vi "Read OOIs.vi"(8 "error in (no error)":errorcluster, 9 "File Path Control":path=path "D:/Espen Tolpinrud/My Documents/LabView/AUR Control System/ROV/Configuration", 10 "ROV Selector":u16(ring) items=["Minerva", "Neptune"], 11 "Vessel In":refnum<class "Vessel.lvclass">) -> (0 "error out":errorcluster, 1 "Observer Names":string[](array[string]), 2 "Controller Names":string[](array[string]), 3 "Vessel Out":refnum<class "Vessel.lvclass">)   [LabVIEW 2012, in "Vessel.lvclass"]
doc: "This method reads a configuration file with a predefined setup in xml. The system is then configured accordingly such that all sensors are initialized, observers and controllers are tuned and all values are given."
uses:
  Vessel.lvclass
  Vessel.lvclass/Vessel.ctl
  <vilib>/LabVIEW Targets/FPGA/cRIO/shared/nicrio_ModuleControls/nicrio_cRIO-9871_FlowControlEnum.ctl
  <vilib>/LabVIEW Targets/FPGA/cRIO/shared/nicrio_ModuleControls/nicrio_cRIO-9871_BaudRateEnum.ctl
  <vilib>/LabVIEW Targets/FPGA/cRIO/shared/nicrio_ModuleControls/nicrio_cRIO-9871_DataBitsEnum.ctl
  <vilib>/LabVIEW Targets/FPGA/cRIO/shared/nicrio_ModuleControls/nicrio_cRIO-9871_ParityEnum.ctl
  <vilib>/LabVIEW Targets/FPGA/cRIO/shared/nicrio_ModuleControls/nicrio_cRIO-9871_StopBitsEnum.ctl
  Observer/Kalman Filter/Kalman Filter.lvclass
  Observer/Attitude Observer/Attitude Observer.lvclass
  Observer/HG Observer/HG Observer.lvclass
  Joystick/Joystick Guidance.lvclass
  Guidance/Altitude Guidance/Altitude Guidance.lvclass
  Guidance/Constant Jerk Guidance/Constant Jerk Guidance.lvclass
  Guidance/CJ Switcher/CJ switcher.lvclass
  Controller/PID Controller/Non Linear PID Controller/Non Linear PID Controller.lvclass
  <vilib>/xml/Load XML File.vi
  Sensor/Sensor(StringArray).vi
  <vilib>/Analysis/Matrix/Numeric/Multiply/Multiply - RM,R.vi
  Observer/Kalman Filter Altitude/Kalman Filter Altitude().vi
  Observer/Kalman Filter/Kalman Filter (Vessel).vi
  Observer/HG Observer/HG Observer().vi
  Joystick/Joystick Guidance ().vi
  Guidance/Constant Jerk Guidance/CJ Guidance().vi
  Controller/PID Controller/Non Linear PID Controller/Non Linear PID Controller().vi
  Thruster/Thruster(ArrayInput).vi
  <resource>/objmgr/DOMUserDefRef.rc
  <vilib>/xml/NI_XML.lvlib
  Sensor/Sensor.lvclass
  Thrust Allocation/Thrust Allocation.lvclass
  Thruster/Thruster.lvclass
  Observer/Kalman Filter Altitude/Kalman Filter Altitude.lvclass
  Controller/Controller.lvclass
  <vilib>/Analysis/Matrix/NI_Matrix.lvlib
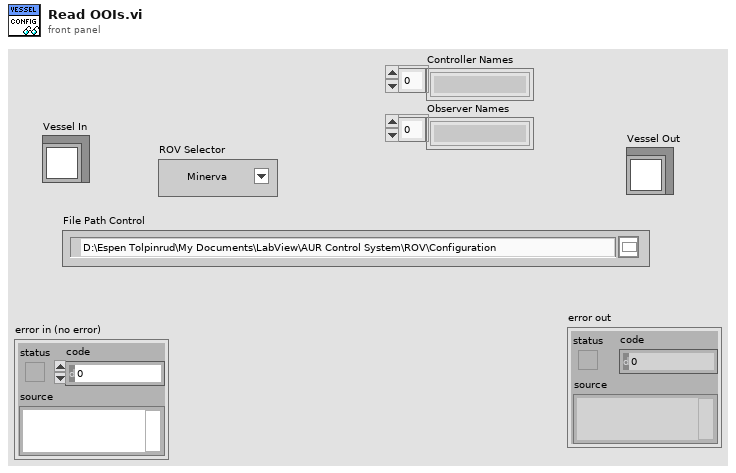
[diagram p1: front panel]
types:
  T1 = typedef "nicrio_cRIO-9871_FlowControlEnum.ctl" = enum8{"None", "Software (XON / XOFF)", "Hardware (RTS / CTS)"}
  T2 = typedef "nicrio_cRIO-9871_StopBitsEnum.ctl" = enum8{"1", "1.5", "2"}
  T3 = typedef "nicrio_cRIO-9871_DataBitsEnum.ctl" = enum8{"5", "6", "7", "8"}
  T4 = typedef "nicrio_cRIO-9871_ParityEnum.ctl" = enum8{"None", "Odd", "Even", "Mark", "Space"}
  T5 = typedef "nicrio_cRIO-9871_BaudRateEnum.ctl" = enum16{"75 bps", "110 bps", "134 bps", "150 bps", "300 bps", "600 bps", "1200 bps", "1800 bps", "2400 bps", "4800 bps", "7200 bps", "9600 bps", "14.4 kbps", "19.2 kbps", "28.8 kbps", "38.4 kbps", "57.6 kbps", "115.2 kbps", "230.4 kbps", "460.8 kbps", "921.6 kbps"}
  T6 = cluster{"Baud Rate":T5, "Data Bits":T3, "Parity":T4, "Stop Bits":T2, "Flow Control":T1}[]
  T7 = cluster{"Baud Rate":T5, "Data Bits":T3, "Parity":T4, "Stop Bits":T2, "Flow Control":T1}
  T8 = typedef "NI_Matrix.lvlib/RealMatrix.ctl" = dbl[][]
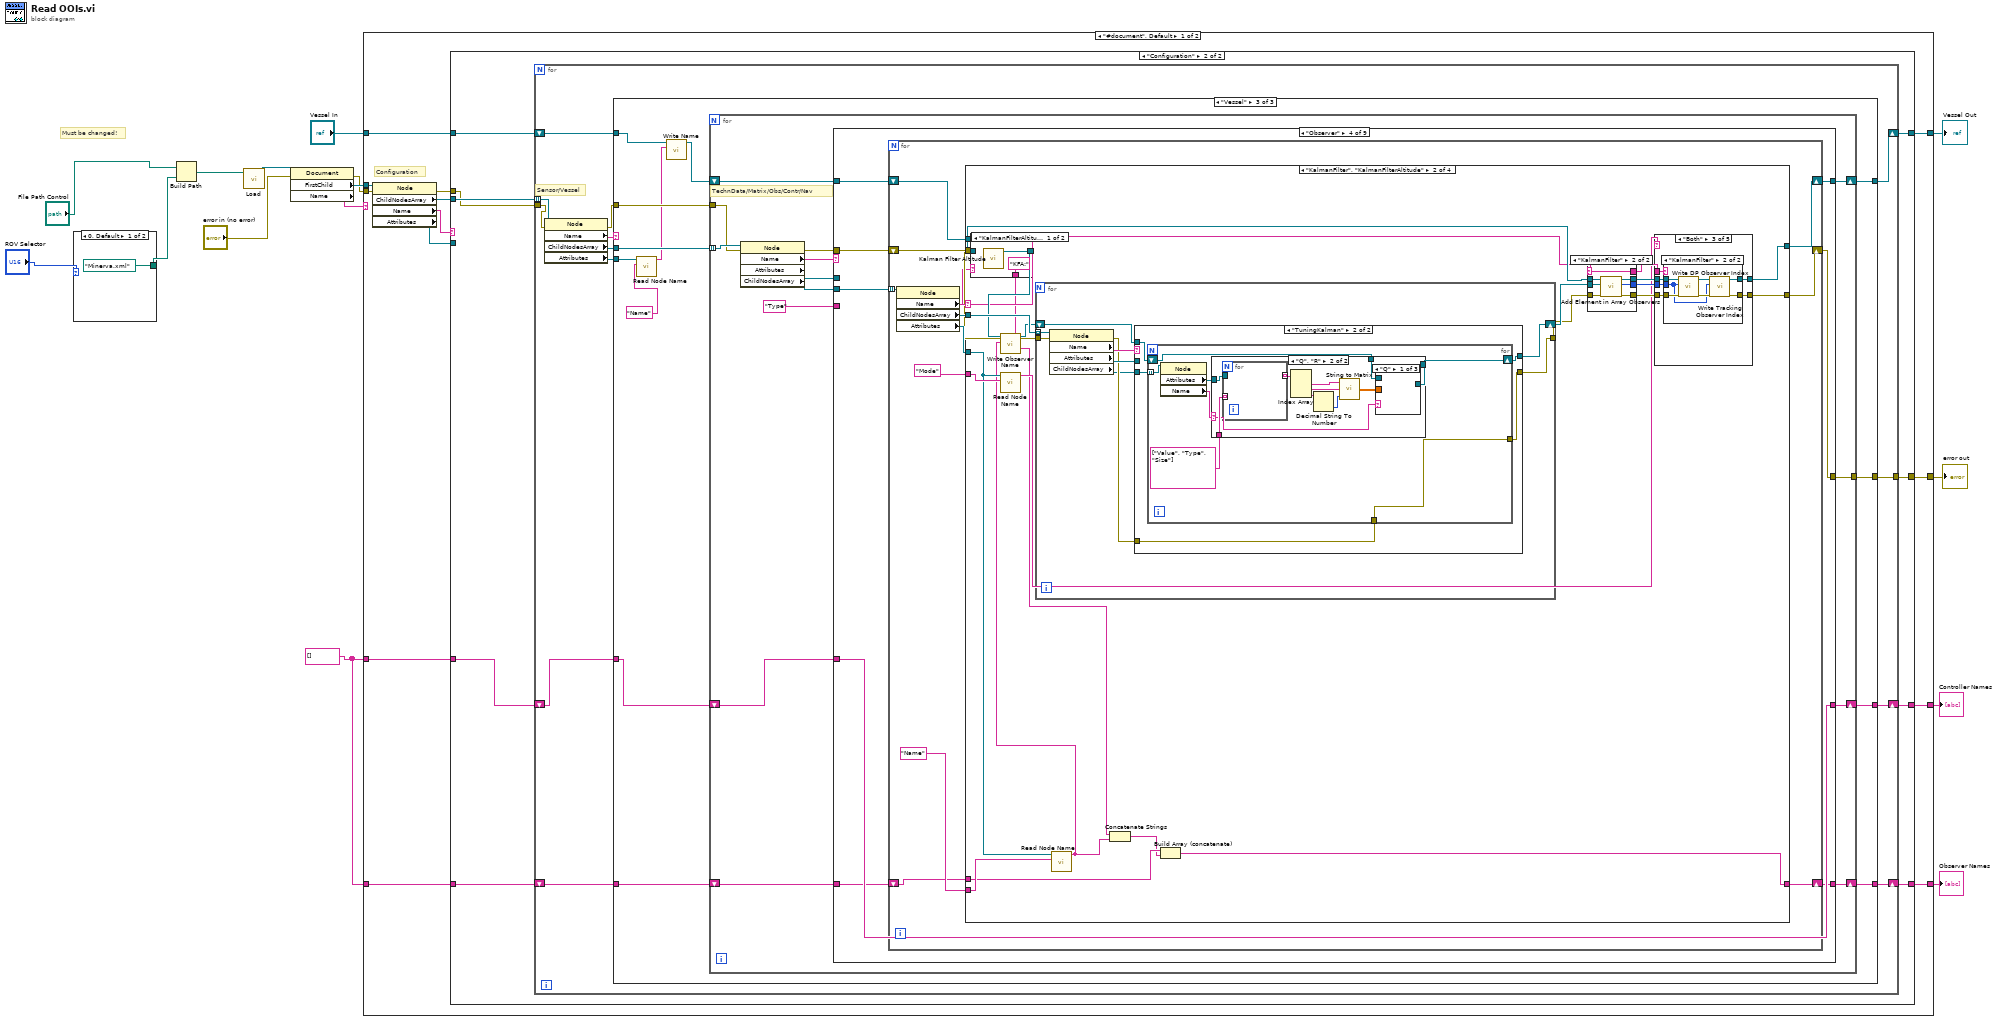
[diagram p0: block diagram]
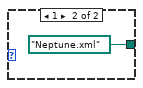
[diagram p2: hidden frame]
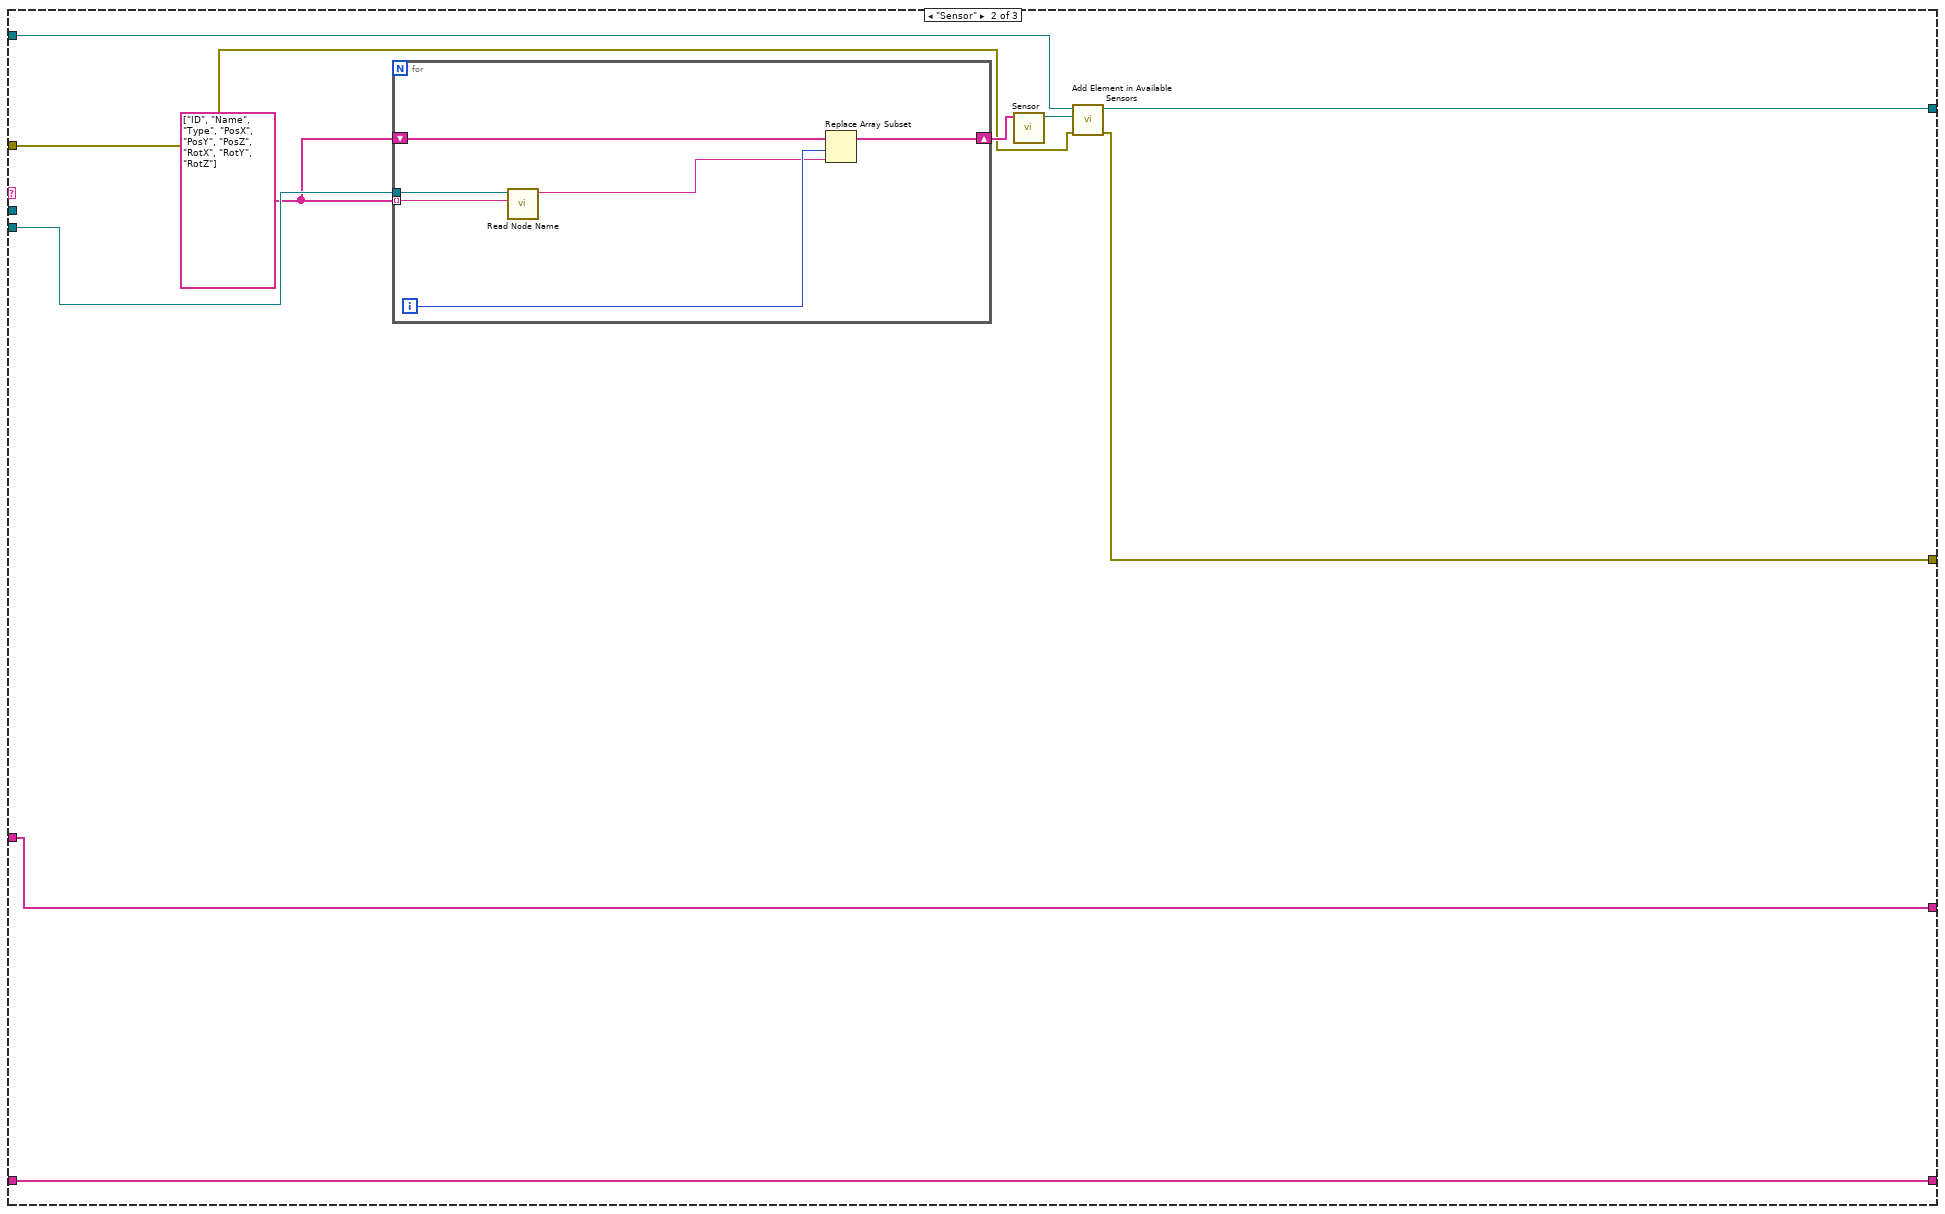
[diagram p5: hidden frame]
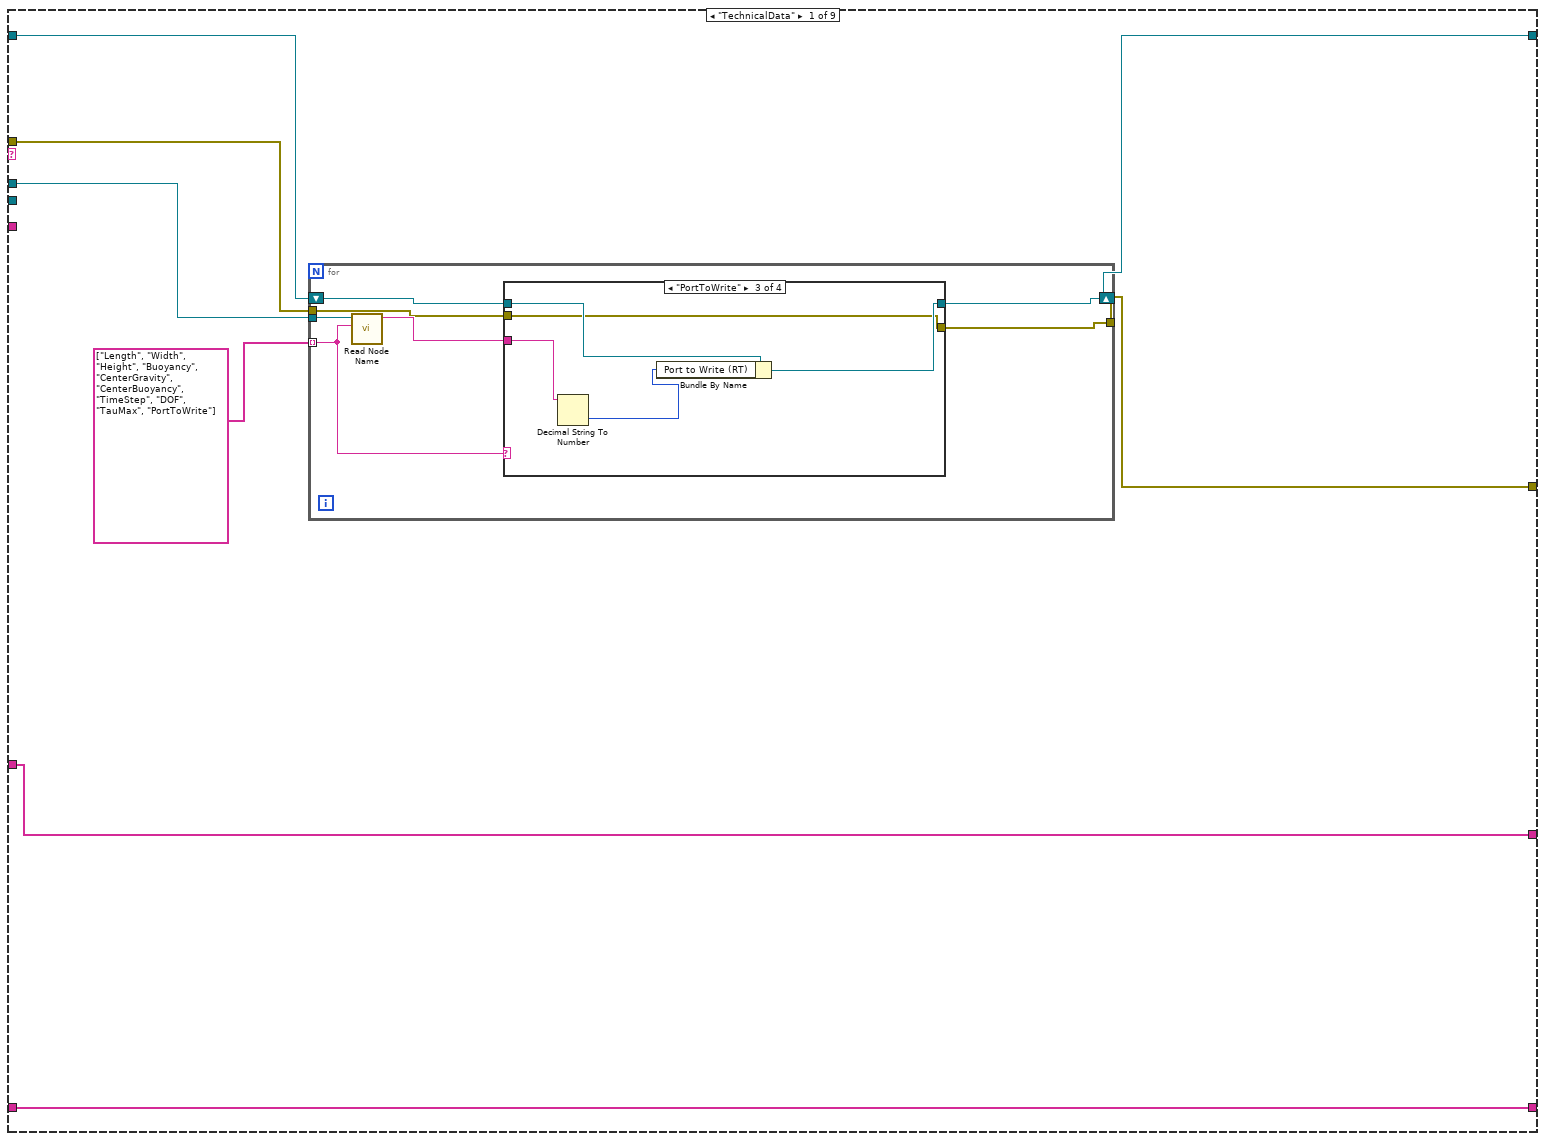
[diagram p6: hidden frame]
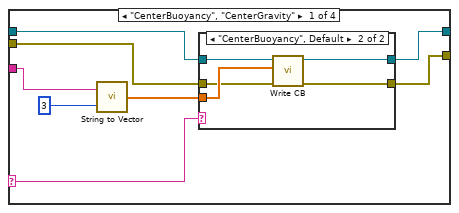
[diagram p7: hidden frame]
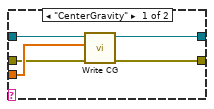
[diagram p8: hidden frame]
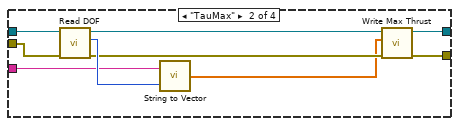
[diagram p9: hidden frame]
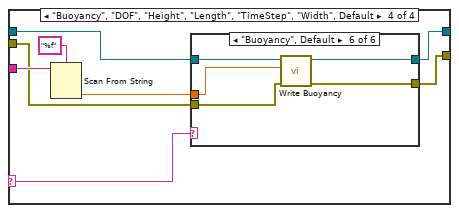
[diagram p10: hidden frame]
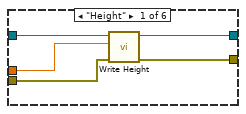
[diagram p11: hidden frame]
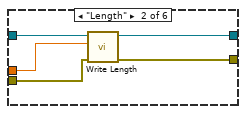
[diagram p12: hidden frame]
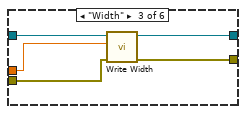
[diagram p13: hidden frame]
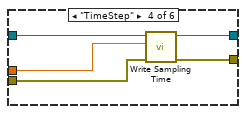
[diagram p14: hidden frame]
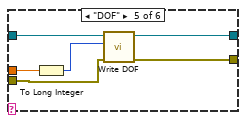
[diagram p15: hidden frame]
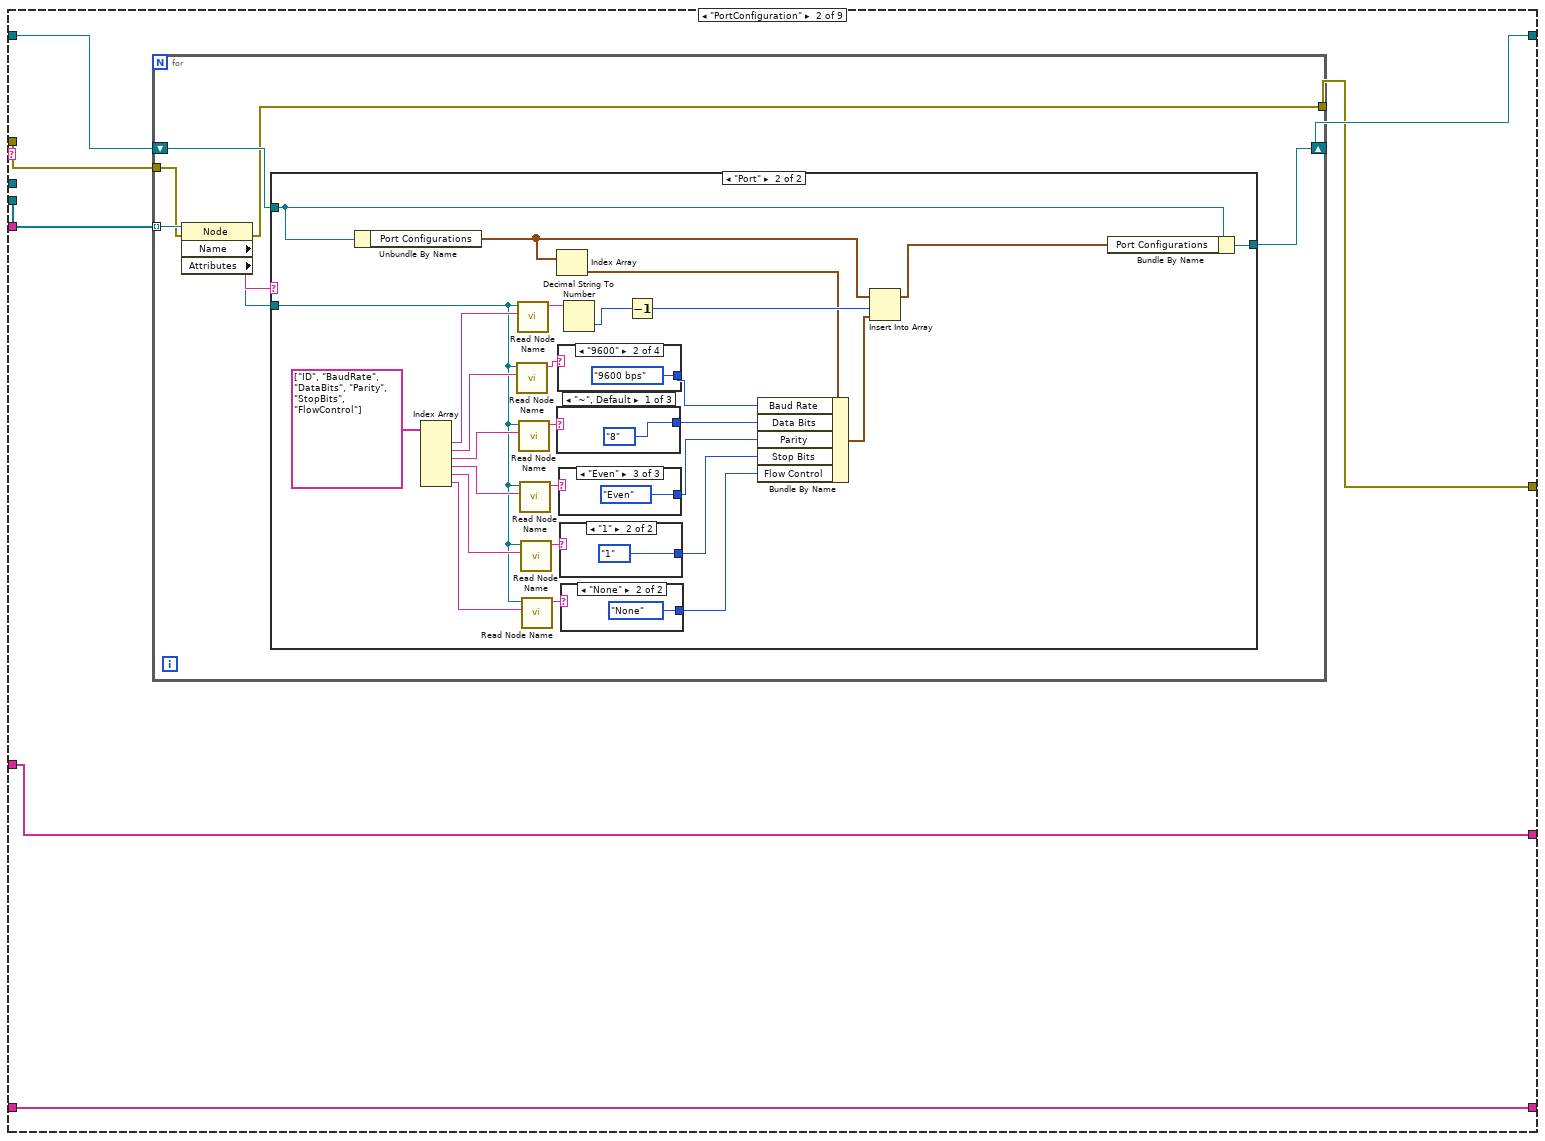
[diagram p16: hidden frame]
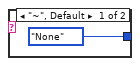
[diagram p18: hidden frame]
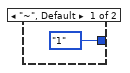
[diagram p19: hidden frame]
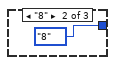
[diagram p20: hidden frame]
diagram:
  w2 = string[] []
  # "Must be changed!"
  n1 = case shown="0, Default" "ROV Selector" {
    tunnel: [path "Minerva.xml" path "Neptune.xml"] -> w6
    frame 0, Default {
    }
    frame 1 {
    }
  }
  n2 = Build Path(base path="File Path Control", name or relative path=w6) -> (appended path=w5:path)
  n3 = call-poly <vilib>:"Load.vi"("path to XML document"=w5) -> ("DOM document out"=w15:refnum<k20>)  [unwired: 12 in, 2 out]
  n4 = property class="Document"(reference=w15, error in="error in (no error)") -> (error out=w10:errorcluster, "FirstChild"=w14:refnum<k20>, "Name"=w13:string)  [unwired: 1 out]
  n5 = case shown="\"#document\", Default" w13 {
    tunnel: w14 -> [w30 _]
    tunnel: "Vessel In" -> [w26 w1002]
    tunnel: [w25 w1002] -> w11
    tunnel: w10 -> [w24 w1001]
    tunnel: [w22 w1001] -> w8
    tunnel: [w21 w1000] -> w3
    tunnel: w2 -> [w20 w1000]
    tunnel: w2 -> [w19 w999]
    tunnel: [w18 w999] -> w1
    frame "#document", Default {
      # "Configuration"
      n6 = property class="Node"(reference=w30, error in=w24) -> (error out=w23:errorcluster, "ChildNodesArray"=w27:refnum<k20>[], "Name"=w28:string, "Attributes"=w29:refnum<k20>)  [unwired: 1 out]
      n7 = case shown="\"Configuration\"" w28 {
        tunnel: w29 -> [_ _]
        tunnel: w27 -> [_ w43]
        tunnel: w26 -> [w34 w42]
        tunnel: [w34 w41] -> w25
        tunnel: w23 -> [w33 w40]
        tunnel: [w33 w39] -> w22
        tunnel: [w32 w38] -> w21
        tunnel: w20 -> [w32 w37]
        tunnel: w19 -> [w31 w36]
        tunnel: [w31 w35] -> w18
        frame "#~", Default {
        }
        frame "Configuration" {
          n8 = for {
            tunnel: w43 -> [w56] mode=indexing
            tunnel: w40 -> [w52]
            tunnel: [w50] -> w39
            shift-right: [w48] -> w41
            shift-left: w42 -> [w49]
            shift-right: [w47] -> w38
            shift-left: w37 -> [w46]
            shift-right: [w44] -> w35
            shift-left: w36 -> [w45]
            # "Sensor/Vessel"
            n9 = property class="Node"(reference=w56, error in=w52) -> (error out=w51:errorcluster, "Name"=w55:string, "ChildNodesArray"=w54:refnum<k20>[], "Attributes"=w53:refnum<k20>)  [unwired: 1 out]
            n10 = case shown="\"Vessel\"" w55 {
              tunnel: w54 -> [_ _ w89]
              tunnel: w53 -> [_ w70 w85]
              tunnel: w49 -> [w60 w67 w83]
              tunnel: [w60 w66 w88] -> w48
              tunnel: w51 -> [w59 w65 w87]
              tunnel: [w59 w63 w86] -> w50
              tunnel: [w58 w62 w80] -> w47
              tunnel: w46 -> [w58 w62 w79]
              tunnel: w45 -> [w57 w61 w78]
              tunnel: [w57 w61 w77] -> w44
              frame "#~", Default {
              }
              frame "Sensor" {
                w64 = string[] ["ID", "Name", "Type", "PosX", "PosY", "PosZ", "RotX", "RotY", "RotZ"]
                n11 = for {
                  tunnel: w64 -> [w73] mode=indexing
                  tunnel: w70 -> [w74]
                  shift-right: [w75] -> w69
                  shift-left: w64 -> [w71]
                  i -> [w76]
                  n12 = call "Read Node Name.vi"("Name"=w73, "Attributes"=w74) -> ("Value"=w72:string)  [unwired: 9 in]
                  n13 = Replace Array Subset(array=w71, new element=w72, index=w76) -> (w75:string[])
                }
                n14 = call-poly "Sensor.vi"("Input"=w69) -> ("Sensor.lvclass"=w68:refnum<class "Sensor.lvclass">)  [unwired: 10 in]
                n15 = call "Add Element in Available Sensors.vi"("error in (no error)"=w65, "Sensor In"=w68, "Vessel in"=w67) -> ("error out"=w63:errorcluster, "Vessel out"=w66:refnum<class "Vessel.lvclass">)  [unwired: 7 in]
              }
              frame "Vessel" {
                n16 = call "Read Node Name.vi"("Name"="Name", "Attributes"=w85) -> ("Value"=w84:string)  [unwired: 9 in]
                n17 = call-dynamic "Write Name.vi"("Name"=w84, "Vessel in"=w83) -> ("Vessel out"=w82:refnum<class "Vessel.lvclass">)  [unwired: 8 in, 1 out]
                n18 = for {
                  tunnel: w89 -> [w103] mode=indexing
                  tunnel: w87 -> [w98]
                  tunnel: [w96] -> w86
                  shift-right: [w95] -> w88
                  shift-left: w82 -> [w94]
                  shift-right: [w93] -> w80
                  shift-left: w79 -> [w92]
                  shift-right: [w90] -> w77
                  shift-left: w78 -> [w91]
                  # "TechnData/Matrix/Obs/Contr/Nav"
                  n19 = property class="Node"(reference=w103, error in=w98) -> (error out=w97:errorcluster, "Name"=w102:string, "Attributes"=w101:refnum<k20>, "ChildNodesArray"=w100:refnum<k20>[])  [unwired: 1 out]
                  n20 = case shown="\"Observer\"" w102 {
                    tunnel: w101 -> [w111 _ _ _ _ w764 w918 w978 _]
                    tunnel: w100 -> [_ w196 w249 w313 w586 w768 _ _ _]
                    tunnel: w94 -> [w109 w195 w252 w310 w584 w767 w915 w972 w998]
                    tunnel: [w108 w194 w251 w311 w583 w763 w917 w971 w998] -> w95
                    tunnel: "Type" -> [_ _ _ _ _ _ w920 _ _]
                    tunnel: w97 -> [w107 w193 w250 w312 w585 w766 w916 w970 w997]
                    tunnel: [w106 w192 w248 w309 w582 w765 w914 w969 w997] -> w96
                    tunnel: [w105 w191 w247 w308 w581 w762 w913 w968 w996] -> w93
                    tunnel: w92 -> [w105 w191 w247 w308 w581 w761 w913 w968 w996]
                    tunnel: w91 -> [w104 w190 w246 w307 w580 w760 w912 w967 w995]
                    tunnel: [w104 w190 w246 w306 w580 w760 w912 w967 w995] -> w90
                    frame "TechnicalData" {
                      n21 = for {
                        tunnel: w111 -> [w118]
                        tunnel: string[] ["Length", "Width", "Height", "Buoyancy", "CenterGravity", "CenterBuoyancy", "TimeStep", "DOF", "TauMax", "PortToWrite"] -> [w117] mode=indexing
                        shift-right: [w114] -> w108
                        shift-left: w109 -> [w115]
                        tunnel: w107 -> [w113]
                        tunnel: [w112] -> w106
                        n22 = call "Read Node Name.vi"("Name"=w117, "Attributes"=w118) -> ("Value"=w116:string)  [unwired: 9 in]
                        n23 = case shown="\"PortToWrite\"" w117 {
                          selector: w117 -> [w126 _ _ w155]
                          tunnel: w116 -> [w123 w141 w149 w158]
                          tunnel: w115 -> [w125 w144 w150 w156]
                          tunnel: [w124 w145 w148 w153] -> w114
                          tunnel: w113 -> [w120 w140 w147 w152]
                          tunnel: [w119 w138 w147 w151] -> w112
                          frame "CenterBuoyancy", "CenterGravity" {
                            n24 = call "String to Vector.vi"("Vector Dimension"=3, "String Input"=w123) -> ("Vector"=w122:dbl[])
                            n25 = case shown="\"CenterBuoyancy\", Default" w126 {
                              tunnel: w125 -> [w131 w136]
                              tunnel: [w130 w135] -> w124
                              tunnel: w122 -> [w129 w134]
                              tunnel: w120 -> [w128 w133]
                              tunnel: [w127 w132] -> w119
                              frame "CenterGravity" {
                                n26 = call "Write CG.vi"("error in (no error)"=w128, "CG"=w129, "Vessel in"=w131) -> ("error out"=w127:errorcluster, "Vessel out"=w130:refnum<class "Vessel.lvclass">)  [unwired: 7 in]
                              }
                              frame "CenterBuoyancy", Default {
                                n27 = call "Write CB.vi"("error in (no error)"=w133, "CB"=w134, "Vessel in"=w136) -> ("error out"=w132:errorcluster, "Vessel out"=w135:refnum<class "Vessel.lvclass">)  [unwired: 7 in]
                              }
                            }
                          }
                          frame "TauMax" {
                            n28 = call-dynamic "Read DOF.vi"("error in (no error)"=w140, "Vessel in"=w144) -> ("error out"=w139:errorcluster, "DOF"=w142:i32, "Vessel out"=w143:refnum<class "Vessel.lvclass">)  [unwired: 7 in]
                            n29 = call "String to Vector.vi"("Vector Dimension"=w142, "String Input"=w141) -> ("Vector"=w137:dbl[])
                            n30 = call "Write Max Thrust.vi"("error in (no error)"=w139, "Max Thrust"=w137, "Vessel in"=w143) -> ("error out"=w138:errorcluster, "Vessel out"=w145:refnum<class "Vessel.lvclass">)  [unwired: 7 in]
                          }
                          frame "PortToWrite" {
                            n31 = Decimal String To Number(string=w149) -> (number=w146:i32)  [unwired: 2 in, 1 out]
                            n32 = Bundle By Name(cluster=w150, "Port to Write (RT)"=w146) -> (w148:refnum<class "Vessel.lvclass">)
                          }
                          frame "Buoyancy", "DOF", "Height", "Length", "TimeStep", "Width", Default {
                            n33 = Scan From String(format string="%f", input string=w158) -> (output 1=w154:dbl)  [unwired: 3 in, 3 out]
                            n34 = case shown="\"Buoyancy\", Default" w155 {
                              tunnel: w156 -> [w163 w168 w173 w178 w184 w189]
                              tunnel: w154 -> [w161 w167 w171 w176 w182 w187]
                              tunnel: [w162 w166 w172 w177 w183 w188] -> w153
                              tunnel: w152 -> [w160 w165 w170 w175 w180 w186]
                              tunnel: [w159 w164 w169 w174 w179 w185] -> w151
                              frame "Height" {
                                n35 = call-dynamic "Write Height.vi"("error in (no error)"=w160, "Height"=w161, "Vessel in"=w163) -> ("error out"=w159:errorcluster, "Vessel out"=w162:refnum<class "Vessel.lvclass">)  [unwired: 7 in]
                              }
                              frame "Length" {
                                n36 = call-dynamic "Write Length.vi"("error in (no error)"=w165, "Length"=w167, "Vessel in"=w168) -> ("error out"=w164:errorcluster, "Vessel out"=w166:refnum<class "Vessel.lvclass">)  [unwired: 7 in]
                              }
                              frame "Width" {
                                n37 = call-dynamic "Write Width.vi"("error in (no error)"=w170, "Width"=w171, "Vessel in"=w173) -> ("error out"=w169:errorcluster, "Vessel out"=w172:refnum<class "Vessel.lvclass">)  [unwired: 7 in]
                              }
                              frame "TimeStep" {
                                n38 = call-dynamic "Write Sampling Time.vi"("error in (no error)"=w175, "Sampling Time"=w176, "Vessel in"=w178) -> ("error out"=w174:errorcluster, "Vessel out"=w177:refnum<class "Vessel.lvclass">)  [unwired: 7 in]
                              }
                              frame "DOF" {
                                n39 = To Long Integer(number=w182) -> (32bit integer=w181:i32)
                                n40 = call-dynamic "Write DOF.vi"("error in (no error)"=w180, "DOF"=w181, "Vessel in"=w184) -> ("error out"=w179:errorcluster, "Vessel out"=w183:refnum<class "Vessel.lvclass">)  [unwired: 7 in]
                              }
                              frame "Buoyancy", Default {
                                n41 = call-dynamic "Write Buoyancy.vi"("error in (no error)"=w186, "Buoyancy"=w187, "Vessel in"=w189) -> ("error out"=w185:errorcluster, "Vessel out"=w188:refnum<class "Vessel.lvclass">)  [unwired: 7 in]
                              }
                            }
                          }
                        }
                      }
                    }
                    frame "PortConfiguration" {
                      n42 = for {
                        tunnel: w196 -> [w203] mode=indexing
                        shift-right: [w199] -> w194
                        shift-left: w195 -> [w200]
                        tunnel: w193 -> [w198]
                        tunnel: [w197] -> w192
                        n43 = property class="Node"(reference=w203, error in=w198) -> (error out=w197:errorcluster, "Name"=w202:string, "Attributes"=w201:refnum<k20>)  [unwired: 1 out]
                        n44 = case shown="\"Port\"" w202 {
                          tunnel: w201 -> [_ w224]
                          tunnel: w200 -> [w204 w217]
                          tunnel: [w204 w215] -> w199
                          frame "#~", Default {
                          }
                          frame "Port" {
                            n45 = Unbundle By Name(w217) -> ("Port Configurations"=w220:T6)
                            n46 = Index Array(array=string[] ["ID", "BaudRate", "DataBits", "Parity", "StopBits", "FlowControl"]) -> (element #1=w230:string, element #2=w229:string, element #3=w228:string, element #4=w227:string, element #5=w226:string, element #6=w225:string)  [unwired: 6 in]
                            n47 = call "Read Node Name.vi"("Name"=w229, "Attributes"=w224) -> ("Value"=w214:string)  [unwired: 9 in]
                            n48 = call "Read Node Name.vi"("Name"=w230, "Attributes"=w224) -> ("Value"=w223:string)  [unwired: 9 in]
                            n49 = call "Read Node Name.vi"("Name"=w228, "Attributes"=w224) -> ("Value"=w210:string)  [unwired: 9 in]
                            n50 = call "Read Node Name.vi"("Name"=w227, "Attributes"=w224) -> ("Value"=w212:string)  [unwired: 9 in]
                            n51 = call "Read Node Name.vi"("Name"=w226, "Attributes"=w224) -> ("Value"=w208:string)  [unwired: 9 in]
                            n52 = call "Read Node Name.vi"("Name"=w225, "Attributes"=w224) -> ("Value"=w206:string)  [unwired: 9 in]
                            n53 = Index Array(array=w220) -> (element=w219:T7)  [unwired: 1 in]
                            n54 = case shown="\"~\", Default" w210 {
                              tunnel: [nicrio_cRIO-9871_DataBitsEnum."8" ("Data Bits") nicrio_cRIO-9871_DataBitsEnum."8" ("Data Bits") nicrio_cRIO-9871_DataBitsEnum."7" ("Data Bits")] -> w209
                              frame "~", Default {
                              }
                              frame "8" {
                              }
                              frame "7" {
                              }
                            }
                            n55 = case shown="\"9600\"" w214 {
                              tunnel: [nicrio_cRIO-9871_BaudRateEnum."57.6 kbps" ("Baud Rate") nicrio_cRIO-9871_BaudRateEnum."9600 bps" ("Baud Rate") nicrio_cRIO-9871_BaudRateEnum."115.2 kbps" ("Baud Rate") nicrio_cRIO-9871_BaudRateEnum."19.2 kbps" ("Baud Rate")] -> w213
                              frame "57.6", Default {
                              }
                              frame "9600" {
                              }
                              frame "115.2" {
                              }
                              frame "19.2" {
                              }
                            }
                            n56 = case shown="\"Even\"" w212 {
                              tunnel: [nicrio_cRIO-9871_ParityEnum."None" ("Parity") nicrio_cRIO-9871_ParityEnum."None" ("Parity") nicrio_cRIO-9871_ParityEnum."Even" ("Parity")] -> w211
                              frame "~", Default {
                              }
                              frame "None" {
                              }
                              frame "Even" {
                              }
                            }
                            n57 = case shown="\"1\"" w208 {
                              tunnel: [nicrio_cRIO-9871_StopBitsEnum."1" ("Stop Bits") nicrio_cRIO-9871_StopBitsEnum."1" ("Stop Bits")] -> w207
                              frame "~", Default {
                              }
                              frame "1" {
                              }
                            }
                            n58 = case shown="\"None\"" w206 {
                              tunnel: [nicrio_cRIO-9871_FlowControlEnum."None" ("Flow Control") nicrio_cRIO-9871_FlowControlEnum."None" ("Flow Control")] -> w205
                              frame "~", Default {
                              }
                              frame "None" {
                              }
                            }
                            n59 = Decimal String To Number(string=w223) -> (number=w222:i32)  [unwired: 2 in, 1 out]
                            n60 = Decrement(x=w222) -> (x-1=w221:i32)
                            n61 = Bundle By Name(cluster=w219, "Baud Rate"=w213, "Data Bits"=w209, "Parity"=w211, "Stop Bits"=w207, "Flow Control"=w205) -> (w218:T7)
                            n62 = Insert Into Array(array=w220, index=w221, new element=w218) -> (w216:T6)
                            n63 = Bundle By Name(cluster=w217, "Port Configurations"=w216) -> (w215:refnum<class "Vessel.lvclass">)
                          }
                        }
                      }
                    }
                    frame "Matrix" {
                      n64 = for {
                        tunnel: w249 -> [w262] mode=indexing
                        tunnel: w250 -> [w259]
                        tunnel: [w258] -> w248
                        shift-right: [w253] -> w251
                        shift-left: w252 -> [w254]
                        n65 = property class="Node"(reference=w262, error in=w259) -> (error out=w255:errorcluster, "Name"=w257:string, "Attributes"=w260:refnum<k20>)  [unwired: 1 out]
                        n66 = case shown="\"AddedMass\", \"Corriolis\", \"LinearDamping\", \"Mass\", \"NonLinearDamping\"" w257 {
                          selector: w257 -> [w264 w271]
                          tunnel: [dbl[][] [] w265] -> w261
                          tunnel: w260 -> [_ w269]
                          tunnel: [w264 w271] -> w256
                          frame "#~", Default {
                          }
                          frame "AddedMass", "Corriolis", "LinearDamping", "Mass", "NonLinearDamping" {
                            n67 = call "Read Node Name.vi"("Name"="Values", "Attributes"=w269) -> ("Value"=w266:string)  [unwired: 9 in]
                            n68 = call "Read Node Name.vi"("Name"="Size", "Attributes"=w269) -> ("Value"=w274:string)  [unwired: 9 in]
                            n69 = call "Read Node Name.vi"("Name"="Type", "Attributes"=w269) -> ("Value"=w268:string)  [unwired: 9 in]
                            n70 = Decimal String To Number(string=w274) -> (number=w267:i32)  [unwired: 2 in, 1 out]
                            n71 = call "String to Matrix.vi"("Matrix Size"=w267, "Matrix Type"=w268, "Value string"=w266) -> ("Output Matrix"=w265:T8)
                          }
                        }
                        n72 = case shown="\"NonLinearDamping\"" w256 {
                          tunnel: w261 -> [_ w278 w286 w293 w296 w303]
                          tunnel: w254 -> [w276 w283 w288 w292 w300 w305]
                          tunnel: [w276 w282 w287 w291 w299 w304] -> w253
                          tunnel: w255 -> [w275 w281 w285 w290 w298 w302]
                          tunnel: [w275 w280 w284 w289 w297 w301] -> w258
                          frame "#~", Default {
                          }
                          frame "Mass" {
                            n73 = call-poly <vilib>:"Multiply.vi"("Real Scalar c"=1, "Real Matrix A"=w278) -> ("A * c"=w277:T8)
                            n74 = call "Write Mass_RB.vi"("error in (no error)"=w281, "Real Matrix"=w277, "Vessel in"=w283) -> ("error out"=w280:errorcluster, "Vessel out"=w282:refnum<class "Vessel.lvclass">)  [unwired: 7 in]
                          }
                          frame "AddedMass" {
                            n75 = call "Write Mass_A.vi"("error in (no error)"=w285, "Real Matrix"=w286, "Vessel in"=w288) -> ("error out"=w284:errorcluster, "Vessel out"=w287:refnum<class "Vessel.lvclass">)  [unwired: 7 in]
                          }
                          frame "LinearDamping" {
                            n76 = call "Write Linear Damping.vi"("error in (no error)"=w290, "Real Matrix"=w293, "Vessel in"=w292) -> ("error out"=w289:errorcluster, "Vessel out"=w291:refnum<class "Vessel.lvclass">)  [unwired: 7 in]
                          }
                          frame "NonLinearDamping" {
                            n77 = call-poly <vilib>:"Multiply.vi"("Real Scalar c"=1, "Real Matrix A"=w296) -> ("A * c"=w294:T8)
                            n78 = call "Write Nonlinear Damping.vi"("error in (no error)"=w298, "Real Matrix"=w294, "Vessel in"=w300) -> ("error out"=w297:errorcluster, "Vessel out"=w299:refnum<class "Vessel.lvclass">)  [unwired: 7 in]
                          }
                          frame "Corriolis" {
                            n79 = call "Write Coriolis_RB.vi"("error in (no error)"=w302, "Real Matrix"=w303, "Vessel in"=w305) -> ("error out"=w301:errorcluster, "Vessel out"=w304:refnum<class "Vessel.lvclass">)  [unwired: 7 in]
                          }
                        }
                      }
                    }
                    frame "Observer" {
                      n80 = for {
                        tunnel: w313 -> [w322] mode=indexing
                        shift-right: [w324] -> w311
                        shift-left: w310 -> [w323]
                        shift-right: [w317] -> w309
                        shift-left: w312 -> [w325]
                        shift-right: [w315] -> w306
                        shift-left: w307 -> [w314]
                        n81 = property class="Node"(reference=w322) -> ("Name"=w321:string, "ChildNodesArray"=w320:refnum<k20>[], "Attributes"=w318:refnum<k20>)  [unwired: 1 in, 2 out]
                        n82 = case shown="\"KalmanFilter\", \"KalmanFilterAltitude\"" w321 {
                          selector: w321 -> [_ w336 _ _]
                          tunnel: w325 -> [w328 w351 w480 w542]
                          tunnel: w323 -> [w327 w346 w481 w545]
                          tunnel: [w327 w348 w479 w544] -> w324
                          tunnel: w320 -> [_ w341 w484 w554]
                          tunnel: "Mode" -> [_ w340 _ _]
                          tunnel: w318 -> [_ w334 w477 w548]
                          tunnel: [w328 w347 w480 w541] -> w317
                          tunnel: "Name" -> [_ w335 w478 w547]
                          tunnel: [w326 w332 w475 w546] -> w315
                          tunnel: w314 -> [w326 w333 w476 w549]
                          frame "#~", Default {
                          }
                          frame "KalmanFilter", "KalmanFilterAltitude" {
                            n83 = case shown="\"KalmanFilterAltitude\", Default" w336 {
                              tunnel: [w423 w426] -> w337
                              tunnel: w346 -> [_ w425]
                              tunnel: ["KFA:" "KFR:"] -> w329
                              frame "KalmanFilterAltitude", Default {
                                n84 = call-poly "Kalman Filter Altitude.vi"() -> ("Kalman Filter Altitude Out"=w423:refnum<class "Kalman Filter Altitude.lvclass">)  [unwired: 11 in]
                              }
                              frame "KalmanFilter" {
                                n85 = call-poly "Kalman Filter.vi"("Vessel.lvclass"=w425) -> ("Observer Library.lvlib:Kalman Filter.lvclass"=w426:refnum<class "Kalman Filter.lvclass">)  [unwired: 10 in]
                              }
                            }
                            n86 = call "Read Node Name.vi"("Name"=w340, "Attributes"=w334) -> ("Value"=w339:string)  [unwired: 9 in]
                            n87 = call "Read Node Name.vi"("Name"=w335, "Attributes"=w334) -> ("Value"=w331:string)  [unwired: 9 in]
                            n88 = call-dynamic "Write Observer Name.vi"("Observer Name"=w331, "Observer in"=w337) -> ("Observer out"=w338:refnum<class "Kalman Filter.lvclass">)  [unwired: 8 in, 1 out]
                            n89 = for {
                              tunnel: w341 -> [w435] mode=indexing
                              tunnel: [w428] -> w349
                              tunnel: w351 -> [w432]
                              shift-right: [w431] -> w350
                              shift-left: w338 -> [w430]
                              n90 = property class="Node"(reference=w435, error in=w432) -> (error out=w429:errorcluster, "Name"=w434:string, "Attributes"=w433:refnum<k20>, "ChildNodesArray"=w427:refnum<k20>[])  [unwired: 1 out]
                              n91 = case shown="\"TuningKalman\"" w434 {
                                tunnel: w433 -> [_ _]
                                tunnel: [w437 w439] -> w431
                                tunnel: w430 -> [w437 w440]
                                tunnel: w429 -> [w436 w442]
                                tunnel: [w436 w438] -> w428
                                tunnel: w427 -> [_ w441]
                                frame "#~", Default {
                                (unwired) FALSE
                                }
                                frame "TuningKalman" {
                                n92 = for {
                                tunnel: w442 -> [w445]
                                tunnel: w441 -> [w449] mode=indexing
                                shift-right: [w443] -> w439
                                shift-left: w440 -> [w446]
                                tunnel: [w445] -> w438
                                n93 = property class="Node"(reference=w449) -> ("Attributes"=w448:refnum<k20>, "Name"=w444:string)  [unwired: 1 in, 2 out]
                                n94 = case shown="\"Q\", \"R\"" w444 {
                                selector: w444 -> [_ w452]
                                tunnel: w448 -> [_ w456]
                                tunnel: string[] ["Value", "Type", "Size"] -> [_ w455]
                                tunnel: w446 -> [w450 w454]
                                tunnel: [w450 w453] -> w443
                                frame "#~", Default {
                                }
                                frame "Q", "R" {
                                n95 = for {
                                tunnel: w456 -> [w471]
                                tunnel: [w470] -> w461 mode=indexing
                                tunnel: w455 -> [w469] mode=indexing
                                n96 = call "Read Node Name.vi"("Name"=w469, "Attributes"=w471) -> ("Value"=w470:string)  [unwired: 9 in]
                                }
                                n97 = Index Array(array=w461) -> (element #1=w457:string, element #2=w458:string, element #3=w459:string)  [unwired: 3 in]
                                n98 = Decimal String To Number(string=w459) -> (number=w460:i32)  [unwired: 2 in, 1 out]
                                n99 = call "String to Matrix.vi"("Matrix Size"=w460, "Matrix Type"=w458, "Value string"=w457) -> ("Output Matrix"=w451:T8)
                                n100 = case shown="\"Q\"" w452 {
                                tunnel: w454 -> [w463 w467 w468]
                                tunnel: [w464 w466 w468] -> w453
                                tunnel: w451 -> [w462 w465 _]
                                frame "Q" {
                                n101 = call-dynamic "Write Q.vi"("Real Matrix"=w462, "Kalman Filter in"=w463) -> ("Kalman Filter out"=w464:refnum<class "Kalman Filter.lvclass">)  [unwired: 8 in, 1 out]
                                }
                                frame "R" {
                                n102 = call-dynamic "Write R.vi"("Real Matrix"=w465, "Kalman Filter in"=w467) -> ("Kalman Filter out"=w466:refnum<class "Kalman Filter.lvclass">)  [unwired: 8 in, 1 out]
                                }
                                frame "#~", Default {
                                }
                                }
                                }
                                }
                                }
                                }
                              }
                            }
                            n103 = Concatenate Strings(w329, w331) -> (w330:string)
                            n104 = Build Array (concatenate)(w333, w330) -> (w332:string[])
                            n105 = case shown="\"KalmanFilter\"" w336 {
                              selector: w336 -> [w352 w359]
                              tunnel: [w353 w365] -> w345
                              tunnel: [w355 w364] -> w344
                              tunnel: [w357 w363] -> w343
                              tunnel: w346 -> [w358 w362]
                              tunnel: w350 -> [w356 w361]
                              tunnel: w349 -> [w354 w360]
                              tunnel: [w352 w359] -> w342
                              frame "KalmanFilterAltitude", Default {
                                n106 = call "Add Element in Array Altitude Observers.vi"("error in (no error)"=w354, "Observer input"=w356, "Vessel in"=w358) -> ("error out"=w353:errorcluster, "Index"=w355:i32, "Vessel out"=w357:refnum<class "Vessel.lvclass">)  [unwired: 6 in]
                              }
                              frame "KalmanFilter" {
                                n107 = call "Add Element in Array Observers.vi"("error in (no error)"=w360, "Observer input"=w361, "Vessel in"=w362) -> ("error out"=w365:errorcluster, "Index"=w364:i32, "Vessel out"=w363:refnum<class "Vessel.lvclass">)  [unwired: 6 in]
                              }
                            }
                            n108 = case shown="\"Both\"" w339 {
                              tunnel: [w370 w382 w388 w404 w407] -> w347
                              tunnel: [w371 w383 w389 w405 w408] -> w348
                              tunnel: w345 -> [w367 w382 w387 w404 w409]
                              tunnel: w344 -> [w368 _ w385 _ w410]
                              tunnel: w343 -> [w369 w383 w386 w405 w411]
                              tunnel: w342 -> [w366 _ w384 _ w406]
                              frame "DP" {
                                n109 = case shown="\"KalmanFilter\"" w366 {
                                tunnel: [w375 w381] -> w371
                                tunnel: [w374 w380] -> w370
                                tunnel: w369 -> [w376 w379]
                                tunnel: w368 -> [w372 w378]
                                tunnel: w367 -> [w373 w377]
                                frame "KalmanFilterAltitude", Default {
                                n110 = call-dynamic "Write DP Altitude Observer Index.vi"("error in (no error)"=w373, "DP Altitude Observer Index"=w372, "Vessel in"=w376) -> ("error out"=w374:errorcluster, "Vessel out"=w375:refnum<class "Vessel.lvclass">)  [unwired: 7 in]
                                }
                                frame "KalmanFilter" {
                                n111 = call-dynamic "Write DP Observer Index.vi"("error in (no error)"=w377, "DP Observer Index"=w378, "Vessel in"=w379) -> ("error out"=w380:errorcluster, "Vessel out"=w381:refnum<class "Vessel.lvclass">)  [unwired: 7 in]
                                }
                                }
                              }
                              frame "#~", Default {
                              }
                              frame "Both" {
                                n112 = case shown="\"KalmanFilter\"" w384 {
                                tunnel: [w394 w403] -> w389
                                tunnel: [w393 w402] -> w388
                                tunnel: w387 -> [w392 w399]
                                tunnel: w386 -> [w396 w398]
                                tunnel: w385 -> [w390 w397]
                                frame "KalmanFilterAltitude", Default {
                                n113 = call-dynamic "Write Tracking Altitude Observer Index.vi"("error in (no error)"=w392, "Tracking Altitude Observer Index"=w390, "Vessel in"=w396) -> ("error out"=w391:errorcluster, "Vessel out"=w395:refnum<class "Vessel.lvclass">)  [unwired: 7 in]
                                n114 = call-dynamic "Write DP Altitude Observer Index.vi"("error in (no error)"=w391, "DP Altitude Observer Index"=w390, "Vessel in"=w395) -> ("error out"=w393:errorcluster, "Vessel out"=w394:refnum<class "Vessel.lvclass">)  [unwired: 7 in]
                                }
                                frame "KalmanFilter" {
                                n115 = call-dynamic "Write DP Observer Index.vi"("error in (no error)"=w399, "DP Observer Index"=w397, "Vessel in"=w398) -> ("error out"=w400:errorcluster, "Vessel out"=w401:refnum<class "Vessel.lvclass">)  [unwired: 7 in]
                                n116 = call-dynamic "Write Tracking Observer Index.vi"("error in (no error)"=w400, "Tracking Observer Index"=w397, "Vessel in"=w401) -> ("error out"=w402:errorcluster, "Vessel out"=w403:refnum<class "Vessel.lvclass">)  [unwired: 7 in]
                                }
                                }
                              }
                              frame "~" {
                              }
                              frame "Tracking" {
                                n117 = case shown="\"KalmanFilterAltitude\", Default" w406 {
                                tunnel: w411 -> [w416 w421]
                                tunnel: w410 -> [w412 w420]
                                tunnel: w409 -> [w413 w419]
                                tunnel: [w415 w418] -> w408
                                tunnel: [w414 w417] -> w407
                                frame "KalmanFilterAltitude", Default {
                                n118 = call-dynamic "Write Tracking Altitude Observer Index.vi"("error in (no error)"=w413, "Tracking Altitude Observer Index"=w412, "Vessel in"=w416) -> ("error out"=w414:errorcluster, "Vessel out"=w415:refnum<class "Vessel.lvclass">)  [unwired: 7 in]
                                }
                                frame "KalmanFilter" {
                                n119 = call-dynamic "Write Tracking Observer Index.vi"("error in (no error)"=w419, "Tracking Observer Index"=w420, "Vessel in"=w421) -> ("error out"=w417:errorcluster, "Vessel out"=w418:refnum<class "Vessel.lvclass">)  [unwired: 7 in]
                                }
                                }
                              }
                            }
                          }
                          frame "Attitude" {
                            n120 = call "Read Node Name.vi"("Name"=w478, "Attributes"=w477) -> ("Value"=w473:string)  [unwired: 9 in]
                            n121 = call "Attitude Observer().vi"("Name"=w473) -> ("Attitude Observer Out"=w483:refnum<class "Attitude Observer.lvclass">)  [unwired: 10 in]
                            n122 = for {
                              tunnel: w484 -> [w491] mode=indexing
                              shift-right: [w485] -> w482
                              shift-left: w483 -> [w486]
                              n123 = property class="Node"(reference=w491) -> ("Name"=w490:string, "ChildNodesArray"=w489:refnum<k20>[], "Attributes"=w488:refnum<k20>)  [unwired: 1 in, 2 out]
                              n124 = case shown="\"TuningAttitude\"" w490 {
                                tunnel: w489 -> [_ _ _ w509]
                                tunnel: w488 -> [_ w499 w504 _]
                                tunnel: "Value" -> [_ w498 w503 _]
                                tunnel: w486 -> [w492 w495 w501 w508]
                                tunnel: [w492 w493 w500 w507] -> w485
                                frame "#~", Default {
                                }
                                frame "Offset" {
                                n125 = call "Read Node Name.vi"("Name"=w498, "Attributes"=w499) -> ("Value"=w497:string)  [unwired: 9 in]
                                n126 = call "String to Vector.vi"("Vector Dimension"=3, "String Input"=w497) -> ("Vector"=w494:dbl[])
                                n127 = call-dynamic "Write MTi Theta Offset.vi"("MTi Theta Offset"=w494, "Attitude Observer in"=w495) -> ("Attitude Observer out"=w493:refnum<class "Attitude Observer.lvclass">)  [unwired: 8 in, 1 out]
                                }
                                frame "MagneticNorth" {
                                n128 = call "Read Node Name.vi"("Name"=w503, "Attributes"=w504) -> ("Value"=w506:string)  [unwired: 9 in]
                                n129 = call "String to Vector.vi"("Vector Dimension"=3, "String Input"=w506) -> ("Vector"=w502:dbl[])
                                n130 = call-dynamic "Write Magnet North.vi"("Magnet North"=w502, "Attitude Observer in"=w501) -> ("Attitude Observer out"=w500:refnum<class "Attitude Observer.lvclass">)  [unwired: 8 in, 1 out]
                                }
                                frame "TuningAttitude" {
                                n131 = for {
                                tunnel: w509 -> [w514] mode=indexing
                                shift-right: [w511] -> w507
                                shift-left: w508 -> [w512]
                                n132 = property class="Node"(reference=w514) -> ("Name"=w510:string, "Attributes"=w513:refnum<k20>)  [unwired: 1 in, 2 out]
                                n133 = case shown="\"KI\", \"KP\"" w510 {
                                selector: w510 -> [_ w516]
                                tunnel: w513 -> [_ w523]
                                tunnel: w512 -> [w515 w518]
                                tunnel: [w515 w517] -> w511
                                frame "#~", Default {
                                }
                                frame "KI", "KP" {
                                n134 = call "Read Node Name.vi"("Name"="Type", "Attributes"=w523) -> ("Value"=w526:string)  [unwired: 9 in]
                                n135 = call "Read Node Name.vi"("Name"="Value", "Attributes"=w523) -> ("Value"=w520:string)  [unwired: 9 in]
                                n136 = call "Read Node Name.vi"("Name"="Size", "Attributes"=w523) -> ("Value"=w522:string)  [unwired: 9 in]
                                n137 = Decimal String To Number(string=w522) -> (number=w521:i32)  [unwired: 2 in, 1 out]
                                n138 = case shown="\"Diag\"" w526 {
                                tunnel: w521 -> [w530 w533]
                                tunnel: [w529 w532] -> w519
                                tunnel: w520 -> [w528 w531]
                                frame "Norm", Default {
                                n139 = call "String to Matrix (Norm).vi"("Martix Dimension"=w530, "String"=w528) -> ("Output Matrix"=w529:T8)
                                }
                                frame "Diag" {
                                n140 = call "String to Matrix (Diag).vi"("Martix Dimension"=w533, "String Input"=w531) -> ("Matrix Out"=w532:T8)
                                }
                                }
                                n141 = case shown="\"KP\"" w516 {
                                tunnel: w519 -> [_ w537 w540]
                                tunnel: w518 -> [w534 w536 w539]
                                tunnel: [w534 w535 w538] -> w517
                                frame "#~", Default {
                                }
                                frame "KP" {
                                n142 = call-dynamic "Write Kp.vi"("Real Matrix"=w537, "Attitude Observer in"=w536) -> ("Attitude Observer out"=w535:refnum<class "Attitude Observer.lvclass">)  [unwired: 8 in, 1 out]
                                }
                                frame "KI" {
                                n143 = call-dynamic "Write Ki.vi"("Real Matrix"=w540, "Attitude Observer in"=w539) -> ("Attitude Observer out"=w538:refnum<class "Attitude Observer.lvclass">)  [unwired: 8 in, 1 out]
                                }
                                }
                                }
                                }
                                }
                                }
                              }
                            }
                            n144 = Concatenate Strings("ATT:", w473) -> (w472:string)
                            n145 = Build Array (concatenate)(w476, w472) -> (w475:string[])
                            n146 = call-dynamic "Add Element in Array Attitude Observer.vi"("Observer in"=w482, "Vessel in"=w481) -> ("Vessel out"=w479:refnum<class "Vessel.lvclass">)  [unwired: 7 in, 2 out]
                          }
                          frame "HGObserver" {
                            n147 = call-poly "HG Observer.vi"() -> ("Observer Library.lvlib:HG Observer.lvclass"=w553:refnum<class "HG Observer.lvclass">)  [unwired: 11 in]
                            n148 = call "Read Node Name.vi"("Name"=w547, "Attributes"=w548) -> ("Value"=w551:string)  [unwired: 9 in]
                            n149 = Concatenate Strings("HGO:", w551) -> (w550:string)
                            n150 = for {
                              tunnel: w554 -> [w561] mode=indexing
                              shift-right: [w555] -> w543
                              shift-left: w553 -> [w556]
                              tunnel: w542 -> [_]
                              n151 = property class="Node"(reference=w561) -> ("Name"=w560:string, "ChildNodesArray"=w559:refnum<k20>[], "Attributes"=w558:refnum<k20>)  [unwired: 1 in, 2 out]
                              n152 = case shown="\"TuningHG\"" w560 {
                                tunnel: w559 -> [_ w565]
                                tunnel: w558 -> [_ _]
                                tunnel: "Value" -> [_ _]
                                tunnel: w556 -> [w562 w564]
                                tunnel: [w562 w563] -> w555
                                frame "#~", Default {
                                }
                                frame "TuningHG" {
                                n153 = for {
                                tunnel: w565 -> [w570] mode=indexing
                                shift-right: [w567] -> w563
                                shift-left: w564 -> [w568]
                                n154 = property class="Node"(reference=w570) -> ("Name"=w566:string, "Attributes"=w569:refnum<k20>)  [unwired: 1 in, 2 out]
                                n155 = case shown="\"Epsilon\"" w566 {
                                tunnel: w569 -> [_ w578]
                                tunnel: w568 -> [w571 w576]
                                tunnel: [w571 w579] -> w567
                                frame "#~", Default {
                                }
                                frame "Epsilon" {
                                n156 = call "Read Node Name.vi"("Name"="Value", "Attributes"=w578) -> ("Value"=w575:string)  [unwired: 9 in]
                                n157 = Search/Split String(string=w575, search string/char (-)=";") -> (substring before match=w573:string)  [unwired: 1 in, 2 out]
                                n158 = Fract/Exp String To Number(string=w573) -> (number=w572:dbl)  [unwired: 3 in, 1 out]
                                n159 = call-dynamic "Write Epsilon.vi"("Epsilon"=w572, "HG Observer in"=w576) -> ("HG Observer out"=w579:refnum<class "HG Observer.lvclass">)  [unwired: 8 in, 1 out]
                                }
                                }
                                }
                                }
                              }
                            }
                            n160 = Build Array (concatenate)(w549, w550) -> (w546:string[])
                            n161 = call "Add Element in Array Observers.vi"("error in (no error)"=w542, "Observer input"=w543, "Vessel in"=w545) -> ("error out"=w541:errorcluster, "Vessel out"=w544:refnum<class "Vessel.lvclass">)  [unwired: 6 in, 1 out]
                          }
                        }
                      }
                    }
                    frame "Navigation" {
                      n162 = for {
                        tunnel: w586 -> [w595] mode=indexing
                        tunnel: w585 -> [w594]
                        tunnel: [w591] -> w582
                        shift-right: [w587] -> w583
                        shift-left: w584 -> [w588]
                        n163 = property class="Node"(reference=w595, error in=w594) -> (error out=w592:errorcluster, "Name"=w593:string, "Attributes"=w590:refnum<k20>, "ChildNodesArray"=w589:refnum<k20>[])  [unwired: 1 out]
                        n164 = case shown="\"Altitude\"" w593 {
                          tunnel: w592 -> [w596 w606 w639 w707 w745]
                          tunnel: [w596 w607 w638 w705 w737] -> w591
                          tunnel: w590 -> [_ _ _ _ _]
                          tunnel: w589 -> [_ w600 w643 w701 w744]
                          tunnel: w588 -> [w597 w605 w642 w708 w746]
                          tunnel: [w597 w604 w640 w706 w738] -> w587
                          frame "#~", Default {
                          }
                          frame "Joystick" {
                            n165 = call-poly "Joystick Guidance.vi"() -> ("Guidance Library.lvlib:Joystick Guidance.lvclass"=w599:refnum<class "Joystick Guidance.lvclass">)  [unwired: 11 in]
                            n166 = for {
                              tunnel: w600 -> [w614] mode=indexing
                              shift-right: [w610] -> w598
                              shift-left: w599 -> [w612]
                              n167 = property class="Node"(reference=w614) -> ("Name"=w613:string, "Attributes"=w611:refnum<k20>)  [unwired: 1 in, 2 out]
                              n168 = case shown="\"Delta\"" w613 {
                                tunnel: w612 -> [w615 w621 w629]
                                tunnel: w611 -> [_ w622 w632]
                                tunnel: [w615 w620 w627] -> w610
                                tunnel: "Value" ("Name") -> [_ w617 w630]
                                tunnel: "Size" -> [_ w616 w631]
                                frame "#~", Default {
                                }
                                frame "Omega" {
                                n169 = call "Read Node Name.vi"("Name"=w617, "Attributes"=w622) -> ("Value"=w626:string)  [unwired: 9 in]
                                n170 = call "Read Node Name.vi"("Name"=w616, "Attributes"=w622) -> ("Value"=w625:string)  [unwired: 9 in]
                                n171 = Scan From String(format string="%d", input string=w625) -> (output 1=w623:i32)  [unwired: 3 in, 3 out]
                                n172 = call "String to Vector.vi"("Vector Dimension"=w623, "String Input"=w626) -> ("Vector"=w619:dbl[])
                                n173 = Build Array(w619) -> (w618:T8)
                                n174 = call-dynamic "Write Omega.vi"("Real Matrix"=w618, "Guidance in"=w621) -> ("Guidance out"=w620:refnum<class "Joystick Guidance.lvclass">)  [unwired: 8 in, 1 out]
                                }
                                frame "Delta" {
                                n175 = call "Read Node Name.vi"("Name"=w630, "Attributes"=w632) -> ("Value"=w637:string)  [unwired: 9 in]
                                n176 = call "Read Node Name.vi"("Name"=w631, "Attributes"=w632) -> ("Value"=w636:string)  [unwired: 9 in]
                                n177 = Scan From String(format string="%d", input string=w636) -> (output 1=w634:i32)  [unwired: 3 in, 3 out]
                                n178 = call "String to Vector.vi"("Vector Dimension"=w634, "String Input"=w637) -> ("Vector"=w633:dbl[])
                                n179 = Build Array(w633) -> (w628:T8)
                                n180 = call-dynamic "Write Delta.vi"("Real Matrix"=w628, "Guidance in"=w629) -> ("Guidance out"=w627:refnum<class "Joystick Guidance.lvclass">)  [unwired: 8 in, 1 out]
                                }
                              }
                            }
                            n181 = call "Add Element in Array Guidance.vi"("error in (no error)"=w606, "Guidance input"=w598, "Vessel in"=w605) -> ("error out"=w603:errorcluster, "Index"=w602:i32, "Vessel out"=w601:refnum<class "Vessel.lvclass">)  [unwired: 6 in]
                            n182 = call-dynamic "Write Joystick Guidance Index.vi"("error in (no error)"=w603, "Joystick Guidance Index"=w602, "Vessel in"=w601) -> ("error out"=w607:errorcluster, "Vessel out"=w604:refnum<class "Vessel.lvclass">)  [unwired: 7 in]
                          }
                          frame "Altitude" {
                            n183 = call "Altitude Guidance().vi"() -> ("Altitude Guidance Out"=w644:refnum<class "Altitude Guidance.lvclass">)  [unwired: 11 in]
                            n184 = for {
                              tunnel: w643 -> [w653] mode=indexing
                              shift-right: [w649] -> w641
                              shift-left: w644 -> [w650]
                              tunnel: w639 -> [w647]
                              tunnel: [w645] -> w638
                              n185 = property class="Node"(reference=w653, error in=w647) -> (error out=w646:errorcluster, "Name"=w652:string, "ChildNodesArray"=w651:refnum<k20>[], "Attributes"=w648:refnum<k20>)  [unwired: 1 out]
                              n186 = case shown="\"Tuning\"" w652 {
                                tunnel: w651 -> [_ w660 _]
                                tunnel: w650 -> [w655 w659 w693]
                                tunnel: [w655 w658 w692] -> w649
                                tunnel: w648 -> [_ _ w698]
                                tunnel: w646 -> [w654 w657 w691]
                                tunnel: [w654 w656 w690] -> w645
                                frame "#~", Default {
                                }
                                frame "Tuning" {
                                n187 = for {
                                tunnel: w660 -> [w668] mode=indexing
                                shift-right: [w665] -> w658
                                shift-left: w659 -> [w666]
                                tunnel: w657 -> [w664]
                                tunnel: [w662] -> w656
                                n188 = property class="Node"(reference=w668, error in=w664) -> (error out=w663:errorcluster, "Name"=w661:string, "Attributes"=w667:refnum<k20>)  [unwired: 1 out]
                                n189 = case shown="\"KI\", \"KP\", \"Kff\"" w661 {
                                selector: w661 -> [_ w671]
                                tunnel: w667 -> [_ w679]
                                tunnel: w666 -> [w670 w677]
                                tunnel: [w670 w676] -> w665
                                tunnel: w663 -> [w669 w673]
                                tunnel: [w669 w672] -> w662
                                frame "#~", Default {
                                }
                                frame "KI", "KP", "Kff" {
                                n190 = call "Read Node Name.vi"("Name"="Value", "Attributes"=w679) -> ("Value"=w675:string)  [unwired: 9 in]
                                n191 = Scan From String(input string=w675, error in=w673) -> (error out=w672:errorcluster, output 1=w674:dbl)  [unwired: 3 in, 2 out]
                                n192 = case shown="\"Kff\"" w671 {
                                tunnel: w677 -> [w680 w683 w685 w689]
                                tunnel: [w680 w681 w684 w688] -> w676
                                tunnel: w674 -> [_ w682 w686 w687]
                                frame "#~", Default {
                                }
                                frame "KP" {
                                n193 = call-dynamic "Write K_p.vi"("K_p"=w682, "Altitude Guidance in"=w683) -> ("Altitude Guidance out"=w681:refnum<class "Altitude Guidance.lvclass">)  [unwired: 8 in, 1 out]
                                }
                                frame "KI" {
                                n194 = call-dynamic "Write K_i.vi"("K_i"=w686, "Altitude Guidance in"=w685) -> ("Altitude Guidance out"=w684:refnum<class "Altitude Guidance.lvclass">)  [unwired: 8 in, 1 out]
                                }
                                frame "Kff" {
                                n195 = call-dynamic "Write K_ff.vi"("K_ff"=w687, "Altitude Guidance in"=w689) -> ("Altitude Guidance out"=w688:refnum<class "Altitude Guidance.lvclass">)  [unwired: 8 in, 1 out]
                                }
                                }
                                }
                                }
                                }
                                }
                                frame "Omega" {
                                n196 = call "Read Node Name.vi"("Name"="Value", "Attributes"=w698) -> ("Value"=w696:string)  [unwired: 9 in]
                                n197 = Scan From String(input string=w696, error in=w691) -> (error out=w690:errorcluster, output 1=w695:dbl)  [unwired: 3 in, 2 out]
                                n198 = Build Array(w695) -> (w694:T8)
                                n199 = call-dynamic "Write Omega.vi"("Real Matrix"=w694, "Guidance in"=w693) -> ("Guidance out"=w692:refnum<class "Altitude Guidance.lvclass">)  [unwired: 8 in, 1 out]
                                }
                              }
                            }
                            n200 = call-dynamic "Add Element in Array Altitude Guidance.vi"("Guidance In"=w641, "Vessel in"=w642) -> ("Vessel out"=w640:refnum<class "Vessel.lvclass">)  [unwired: 8 in, 1 out]
                          }
                          frame "ConstantJerk" {
                            n201 = call-poly "CJ Guidance.vi"() -> ("Guidance Library.lvlib:Constant Jerk Guidance.lvclass"=w700:refnum<class "Constant Jerk Guidance.lvclass">)  [unwired: 11 in]
                            n202 = for {
                              tunnel: w701 -> [w715] mode=indexing
                              shift-right: [w711] -> w699
                              shift-left: w700 -> [w713]
                              n203 = property class="Node"(reference=w715) -> ("Name"=w714:string, "Attributes"=w712:refnum<k20>)  [unwired: 1 in, 2 out]
                              n204 = case shown="\"jav_rad\"" w714 {
                                tunnel: w713 -> [w716 w718 w729]
                                tunnel: w712 -> [_ w722 w732]
                                tunnel: [w716 w719 w728] -> w711
                                tunnel: "Value" ("Name") -> [_ w721 w730]
                                tunnel: "Size" -> [_ w720 w731]
                                frame "#~", Default {
                                }
                                frame "jav_pos" {
                                n205 = call "Read Node Name.vi"("Name"=w721, "Attributes"=w722) -> ("Value"=w726:string)  [unwired: 9 in]
                                n206 = call "Read Node Name.vi"("Name"=w720, "Attributes"=w722) -> ("Value"=w725:string)  [unwired: 9 in]
                                n207 = Scan From String(format string="%d", input string=w725) -> (output 1=w723:i32)  [unwired: 3 in, 3 out]
                                n208 = call "String to Vector.vi"("Vector Dimension"=w723, "String Input"=w726) -> ("Vector"=w717:dbl[])
                                n209 = call-dynamic "Write jav pos.vi"("jav pos"=w717, "Constant Jerk Guidance in"=w718) -> ("Constant Jerk Guidance out"=w719:refnum<class "Constant Jerk Guidance.lvclass">)  [unwired: 8 in, 1 out]
                                }
                                frame "jav_rad" {
                                n210 = call "Read Node Name.vi"("Name"=w730, "Attributes"=w732) -> ("Value"=w736:string)  [unwired: 9 in]
                                n211 = call "Read Node Name.vi"("Name"=w731, "Attributes"=w732) -> ("Value"=w735:string)  [unwired: 9 in]
                                n212 = Scan From String(format string="%d", input string=w735) -> (output 1=w733:i32)  [unwired: 3 in, 3 out]
                                n213 = call "String to Vector.vi"("Vector Dimension"=w733, "String Input"=w736) -> ("Vector"=w727:dbl[])
                                n214 = call-dynamic "Write jav rad.vi"("jav rad"=w727, "Constant Jerk Guidance in"=w729) -> ("Constant Jerk Guidance out"=w728:refnum<class "Constant Jerk Guidance.lvclass">)  [unwired: 8 in, 1 out]
                                }
                              }
                            }
                            n215 = call "Add Element in Array Guidance.vi"("error in (no error)"=w707, "Guidance input"=w699, "Vessel in"=w708) -> ("error out"=w702:errorcluster, "Index"=w703:i32, "Vessel out"=w704:refnum<class "Vessel.lvclass">)  [unwired: 6 in]
                            n216 = call-dynamic "Write DP Guidance Index.vi"("error in (no error)"=w702, "DP Guidance Index"=w703, "Vessel in"=w704) -> ("error out"=w705:errorcluster, "Vessel out"=w706:refnum<class "Vessel.lvclass">)  [unwired: 7 in]
                          }
                          frame "CJSwitcher" {
                            n217 = call "CJ switcher().vi"() -> ("Guidance Library.lvlib:CJ switcher.lvclass"=w742:refnum<class "CJ switcher.lvclass">)  [unwired: 11 in]
                            n218 = for {
                              tunnel: w744 -> [w752] mode=indexing
                              shift-right: [w748] -> w743
                              shift-left: w742 -> [w750]
                              n219 = property class="Node"(reference=w752) -> ("Name"=w751:string, "Attributes"=w749:refnum<k20>)  [unwired: 1 in, 2 out]
                              n220 = case shown="\"pause_duration\"" w751 {
                                tunnel: w750 -> [w753 w757]
                                tunnel: w749 -> [_ w759]
                                tunnel: [w753 w756] -> w748
                                tunnel: "Value" ("Name") -> [_ w758]
                                frame "#~", Default {
                                }
                                frame "pause_duration" {
                                n221 = call "Read Node Name.vi"("Name"=w758, "Attributes"=w759) -> ("Value"=w755:string)  [unwired: 9 in]
                                n222 = Scan From String(input string=w755) -> (output 1=w754:dbl)  [unwired: 4 in, 3 out]
                                n223 = call-dynamic "Write pause duration.vi"("pause duration"=w754, "CJ switcher in"=w757) -> ("CJ switcher out"=w756:refnum<class "CJ switcher.lvclass">)  [unwired: 8 in, 1 out]
                                }
                              }
                            }
                            n224 = call "Add Element in Array Guidance.vi"("error in (no error)"=w745, "Guidance input"=w743, "Vessel in"=w746) -> ("error out"=w739:errorcluster, "Index"=w740:i32, "Vessel out"=w741:refnum<class "Vessel.lvclass">)  [unwired: 6 in]
                            n225 = call-dynamic "Write Tracking Guidance Index.vi"("error in (no error)"=w739, "Tracking Guidance Index"=w740, "Vessel in"=w741) -> ("error out"=w737:errorcluster, "Vessel out"=w738:refnum<class "Vessel.lvclass">)  [unwired: 7 in]
                          }
                        }
                      }
                    }
                    frame "Controller" {
                      n226 = for {
                        tunnel: w768 -> [w774] mode=indexing
                        tunnel: w766 -> [w777]
                        tunnel: [w776] -> w765
                        tunnel: w764 -> [_]
                        shift-right: [w775] -> w763
                        shift-left: w767 -> [w778]
                        shift-right: [w770] -> w762
                        shift-left: w761 -> [w769]
                        n227 = property class="Node"(reference=w774) -> ("Name"=w771:string, "ChildNodesArray"=w773:refnum<k20>[], "Attributes"=w772:refnum<k20>)  [unwired: 1 in, 2 out]
                        n228 = case shown="\"LQR\", \"PIDNonLinear\"" w771 {
                          selector: w771 -> [_ w791]
                          tunnel: w774 -> [_ _]
                          tunnel: w778 -> [w780 w795]
                          tunnel: w777 -> [w781 w802]
                          tunnel: [w781 w793] -> w776
                          tunnel: [w780 w794] -> w775
                          tunnel: w773 -> [_ w792]
                          tunnel: w772 -> [_ w788]
                          tunnel: [w779 w787] -> w770
                          tunnel: w769 -> [w779 w786]
                          frame "#~", Default {
                          }
                          frame "LQR", "PIDNonLinear" {
                            n229 = case shown="\"PIDNonLinear\", Default" w791 {
                              tunnel: [w804] -> w790
                              tunnel: ["NLP:"] -> w785
                              frame "PIDNonLinear", Default {
                                n230 = call-poly "Non Linear PID Controller.vi"() -> ("Controller Library:Non Linear PID Controller.lvclass"=w804:refnum<class "Non Linear PID Controller.lvclass">)  [unwired: 11 in]
                              }
                            }
                            n231 = call "Read Node Name.vi"("Name"="Name", "Attributes"=w788) -> ("Value"=w784:string)  [unwired: 9 in]
                            n232 = call "Write Controller Name.vi"("Controller Name"=w784, "Controller in"=w790) -> ("Controller out"=w782:refnum<class "Non Linear PID Controller.lvclass">)  [unwired: 8 in, 1 out]
                            n233 = for {
                              tunnel: w802 -> [w832]
                              tunnel: w791 -> [w828]
                              shift-right: [w826] -> w796
                              shift-left: w782 -> [w827]
                              tunnel: [w825] -> w793
                              tunnel: w792 -> [w824] mode=indexing
                              n234 = property class="Node"(reference=w824, error in=w832) -> (error out=w831:errorcluster, "Name"=w835:string, "Attributes"=w833:refnum<k20>, "ChildNodesArray"=w830:refnum<k20>[])  [unwired: 1 out]
                              n235 = case shown="\"~\", Default" w828 {
                                tunnel: w835 -> [_ w880]
                                tunnel: string[] ["Kanti", "TypeKanti", "SizeKanti", "IntegralLimit"] -> [_ w879]
                                tunnel: w833 -> [_ w878]
                                tunnel: w831 -> [w870 w877]
                                tunnel: w827 -> [w871 w876]
                                tunnel: [w871 w873] -> w829
                                tunnel: [w870 w872] -> w825
                                frame "~", Default {
                                }
                                frame "PIDNonLinear" {
                                # "A safe cast"
                                n236 = To More Specific Class(target class=refnum<class "Non Linear PID Controller.lvclass"> refnum ("Controller Library:Non Linear PID Controller.lvclass"), reference=w876) -> (specific class reference=w875:refnum<class "Non Linear PID Controller.lvclass">)  [unwired: 1 in, 1 out]
                                n237 = case shown="\"SpeedController\"" w880 {
                                tunnel: w879 -> [_ w885 _]
                                tunnel: w878 -> [_ w887 w911]
                                tunnel: w875 -> [w881 w884 w906]
                                tunnel: [w881 w888 w905] -> w873
                                tunnel: w877 -> [w882 w883 w904]
                                tunnel: [w882 w889 w903] -> w872
                                frame "#~", Default {
                                }
                                frame "Tuning" {
                                n238 = Index Array(array=w885) -> (element #1=w902:string, element #2=w901:string, element #3=w900:string, element #4=w899:string)  [unwired: 4 in]
                                n239 = call "Read Node Name.vi"("Name"=w902, "Attributes"=w887) -> ("Value"=w898:string)  [unwired: 9 in]
                                n240 = call "Read Node Name.vi"("Name"=w901, "Attributes"=w887) -> ("Value"=w897:string)  [unwired: 9 in]
                                n241 = call "Read Node Name.vi"("Name"=w900, "Attributes"=w887) -> ("Value"=w896:string)  [unwired: 9 in]
                                n242 = call "Read Node Name.vi"("Name"=w899, "Attributes"=w887) -> ("Value"=w894:string)  [unwired: 9 in]
                                n243 = Decimal String To Number(string=w896) -> (number=w895:i32)  [unwired: 2 in, 1 out]
                                n244 = call "String to Vector.vi"("Vector Dimension"=6, "String Input"=w894) -> ("Vector"=w893:dbl[])
                                n245 = call "String to Matrix.vi"("Matrix Size"=w895, "Matrix Type"=w897, "Value string"=w898) -> ("Output Matrix"=w892:T8)
                                n246 = call-dynamic "Write K_anti.vi"("error in (no error)"=w883, "Real Matrix"=w892, "Non Linear PID Controller in"=w884) -> ("error out"=w890:errorcluster, "Non Linear PID Controller out"=w891:refnum<class "Non Linear PID Controller.lvclass">)  [unwired: 7 in]
                                n247 = call-dynamic "Write Int_limit.vi"("error in (no error)"=w890, "Int_limit"=w893, "Non Linear PID Controller in"=w891) -> ("error out"=w889:errorcluster, "Non Linear PID Controller out"=w888:refnum<class "Non Linear PID Controller.lvclass">)  [unwired: 7 in]
                                }
                                frame "SpeedController" {
                                n248 = call "Read Node Name.vi"("Name"="Value", "Attributes"=w911) -> ("Value"=w909:string)  [unwired: 9 in]
                                n249 = Equal?(x=w909, y="Y") -> (x = y?=w907:bool)
                                n250 = call-dynamic "Write Speed Controller.vi"("error in (no error)"=w904, "Speed Controller"=w907, "Non Linear PID Controller in"=w906) -> ("error out"=w903:errorcluster, "Non Linear PID Controller out"=w905:refnum<class "Non Linear PID Controller.lvclass">)  [unwired: 7 in]
                                }
                                }
                                }
                              }
                              n251 = for {
                                tunnel: w830 -> [w841] mode=indexing
                                shift-right: [w836] -> w826
                                shift-left: w829 -> [w840]
                                n252 = property class="Node" props=["ChildNodesArray", "Attributes", "Name"](reference=w841) -> ("Attributes"=w837:refnum<k20>, "Name"=w839:string)  [unwired: 1 in, 3 out]
                                n253 = case shown="\"KD\", \"KI\", \"KIS\", \"KP\", \"Q\", \"R\"" w839 {
                                selector: w839 -> [_ w843]
                                tunnel: w840 -> [w842 w845]
                                tunnel: string[] ["Value", "Type", "Size"] -> [_ w850]
                                tunnel: w837 -> [_ w849]
                                tunnel: [w842 w844] -> w836
                                frame "#~", Default {
                                }
                                frame "KD", "KI", "KIS", "KP", "Q", "R" {
                                n254 = Index Array(array=w850) -> (element #1=w848:string, element #2=w851:string, element #3=w852:string)  [unwired: 3 in]
                                n255 = call "Read Node Name.vi"("Name"=w848, "Attributes"=w849) -> ("Value"=w847:string)  [unwired: 9 in]
                                n256 = call "Read Node Name.vi"("Name"=w851, "Attributes"=w849) -> ("Value"=w853:string)  [unwired: 9 in]
                                n257 = call "Read Node Name.vi"("Name"=w852, "Attributes"=w849) -> ("Value"=w854:string)  [unwired: 9 in]
                                n258 = Decimal String To Number(string=w854) -> (number=w855:i32)  [unwired: 2 in, 1 out]
                                n259 = call "String to Matrix.vi"("Matrix Size"=w855, "Matrix Type"=w853, "Value string"=w847) -> ("Output Matrix"=w846:T8)
                                n260 = case shown="\"KIS\"" w843 {
                                tunnel: w846 -> [w856 w859 w862 w865]
                                tunnel: w845 -> [w858 w861 w864 w869]
                                tunnel: [w857 w860 w863 w866] -> w844
                                frame "KI", Default {
                                n261 = call-dynamic "Write K_I.vi"("Real Matrix"=w856, "PID Controller in"=w858) -> ("PID Controller out"=w857:refnum<class "Non Linear PID Controller.lvclass">)  [unwired: 8 in, 1 out]
                                }
                                frame "KP" {
                                n262 = call-dynamic "Write K_P.vi"("Real Matrix"=w859, "PID Controller in"=w861) -> ("PID Controller out"=w860:refnum<class "Non Linear PID Controller.lvclass">)  [unwired: 8 in, 1 out]
                                }
                                frame "KD" {
                                n263 = call-dynamic "Write K_D.vi"("Real Matrix"=w862, "PID Controller in"=w864) -> ("PID Controller out"=w863:refnum<class "Non Linear PID Controller.lvclass">)  [unwired: 8 in, 1 out]
                                }
                                frame "KIS" {
                                n264 = To More Specific Class(target class=refnum<class "Non Linear PID Controller.lvclass"> refnum ("Controller Library:Non Linear PID Controller.lvclass"), reference=w869) -> (specific class reference=w867:refnum<class "Non Linear PID Controller.lvclass">)  [unwired: 1 in, 1 out]
                                n265 = call-dynamic "Write KI_speed.vi"("Real Matrix"=w865, "Non Linear PID Controller in"=w867) -> ("Non Linear PID Controller out"=w866:refnum<class "Non Linear PID Controller.lvclass">)  [unwired: 8 in, 1 out]
                                }
                                }
                                }
                                }
                              }
                            }
                            n266 = Concatenate Strings(w785, w784) -> (w783:string)
                            n267 = Build Array (concatenate)(w786, w783) -> (w787:string[])
                            n268 = call "Read Node Name.vi"("Name"="Mode", "Attributes"=w788) -> ("Value"=w797:string)  [unwired: 9 in]
                            n269 = call "Add Element in Array Controllers.vi"("Controller Input"=w796, "Vessel in"=w795) -> ("error out"=w799:errorcluster, "Index"=w801:i32, "Vessel out"=w800:refnum<class "Vessel.lvclass">)  [unwired: 7 in]
                            n270 = case shown="\"Tracking\"" w797 {
                              tunnel: w801 -> [w808 _ w815 w823]
                              tunnel: w800 -> [w809 w810 w816 w822]
                              tunnel: w799 -> [w807 w811 w814 w819]
                              tunnel: [w806 w811 w813 w817] -> _
                              tunnel: [w805 w810 w812 w820] -> w794
                              frame "DP" {
                                n271 = call "Write DP Controller Index.vi"("error in (no error)"=w807, "DP Controller Index"=w808, "Vessel in"=w809) -> ("error out"=w806:errorcluster, "Vessel out"=w805:refnum<class "Vessel.lvclass">)  [unwired: 7 in]
                              }
                              frame "#~", Default {
                              }
                              frame "Tracking" {
                                n272 = call "Write Tracking Controller Index.vi"("error in (no error)"=w814, "Tracking Controller Index"=w815, "Vessel in"=w816) -> ("error out"=w813:errorcluster, "Vessel out"=w812:refnum<class "Vessel.lvclass">)  [unwired: 7 in]
                              }
                              frame "Both" {
                                n273 = call "Write DP Controller Index.vi"("error in (no error)"=w819, "DP Controller Index"=w823, "Vessel in"=w822) -> ("error out"=w818:errorcluster, "Vessel out"=w821:refnum<class "Vessel.lvclass">)  [unwired: 7 in]
                                n274 = call "Write Tracking Controller Index.vi"("error in (no error)"=w818, "Tracking Controller Index"=w823, "Vessel in"=w821) -> ("error out"=w817:errorcluster, "Vessel out"=w820:refnum<class "Vessel.lvclass">)  [unwired: 7 in]
                              }
                            }
                          }
                        }
                      }
                    }
                    frame "Thruster" {
                      n275 = call "Read Node Name.vi"("Name"=w920, "Attributes"=w918) -> ("Value"=w919:string)  [unwired: 9 in]
                      n276 = case shown="\"Fixed\", Default" w919 {
                        selector: w919 -> [w939 _]
                        tunnel: w918 -> [w928 _]
                        tunnel: w915 -> [w934 w966]
                        tunnel: [w940 w966] -> w917
                        tunnel: w916 -> [w931 w965]
                        tunnel: [w935 w965] -> w914
                        frame "Fixed", Default {
                          w921 = 1
                          n277 = call "Read Node Name.vi"("Name"="ID", "Attributes"=w928) -> ("Value"=w956:string)  [unwired: 9 in]
                          n278 = call "Read Node Name.vi"("Name"="PosX", "Attributes"=w928) -> ("Value"=w955:string)  [unwired: 9 in]
                          n279 = call "Read Node Name.vi"("Name"="PosY", "Attributes"=w928) -> ("Value"=w954:string)  [unwired: 9 in]
                          n280 = call "Read Node Name.vi"("Name"="PosZ", "Attributes"=w928) -> ("Value"=w953:string)  [unwired: 9 in]
                          n281 = call "Read Node Name.vi"("Name"="RotTheta", "Attributes"=w928) -> ("Value"=w952:string)  [unwired: 9 in]
                          n282 = call "Read Node Name.vi"("Name"="RotPhi", "Attributes"=w928) -> ("Value"=w951:string)  [unwired: 9 in]
                          n283 = call "Read Node Name.vi"("Name"="Coefficient", "Attributes"=w928) -> ("Value"=w938:string)  [unwired: 9 in]
                          n284 = call "Read Node Name.vi"("Name"="MaxRPM", "Attributes"=w928) -> ("Value"=w950:string)  [unwired: 9 in]
                          n285 = call "Read Node Name.vi"("Name"="Name", "Attributes"=w928) -> ("Value"=w927:string)  [unwired: 9 in]
                          n286 = Fract/Exp String To Number(string=w951) -> (number=w944:dbl)  [unwired: 3 in, 1 out]
                          n287 = Decimal String To Number(string=w956) -> (number=w949:i32)  [unwired: 2 in, 1 out]
                          n288 = Fract/Exp String To Number(string=w955) -> (number=w948:dbl)  [unwired: 3 in, 1 out]
                          n289 = Fract/Exp String To Number(string=w954) -> (number=w947:dbl)  [unwired: 3 in, 1 out]
                          n290 = Fract/Exp String To Number(string=w952) -> (number=w945:dbl)  [unwired: 3 in, 1 out]
                          n291 = Fract/Exp String To Number(string=w953) -> (number=w946:dbl)  [unwired: 3 in, 1 out]
                          n292 = Fract/Exp String To Number(string=w950) -> (number=w926:dbl)  [unwired: 3 in, 1 out]
                          n293 = Scan From String(format string="%f:%f;", input string=w938) -> (output 1=w925:dbl, output 2=w923:dbl)  [unwired: 4 in, 3 out]
                          n294 = call "Read Thrust Allocation.lvclass.vi"("error in (no error)"=w931, "Vessel in"=w934) -> ("error out"=w930:errorcluster, "Thrust Allocation.lvclass"=w932:refnum<class "Thrust Allocation.lvclass">, "Vessel out"=w933:refnum<class "Vessel.lvclass">)  [unwired: 7 in]
                          n295 = Multiply(x=w921, y=w925) -> (x*y=w924:dbl)
                          n296 = Multiply(x=w921, y=w923) -> (x*y=w922:dbl)
                          n297 = Build Array(w948, w947, w946, w945, w944, w924, w922, w926) -> (w943:dbl[])
                          n298 = call-poly "Thruster.vi"("Name"=w927, "Type Input"=w939, "ArrayInput"=w943) -> ("Thruster.lvclass"=w942:refnum<class "Thruster.lvclass">)  [unwired: 8 in]
                          n299 = call "Insert Thruster.vi"("error in (no error)"=w930, "Index"=w949, "Thruster In"=w942, "Thrust Allocation in"=w932) -> ("error out"=w936:errorcluster, "Thrust Allocation out"=w941:refnum<class "Thrust Allocation.lvclass">)  [unwired: 6 in]
                          n300 = call "Write Thrust Allocation.lvclass.vi"("error in (no error)"=w936, "Thrust Allocation.lvclass"=w941, "Vessel in"=w933) -> ("error out"=w935:errorcluster, "Vessel out"=w940:refnum<class "Vessel.lvclass">)  [unwired: 7 in]
                        }
                        frame "Azimuth" {
                        }
                      }
                    }
                    frame "SensorsInstalled" {
                      n301 = call "Read Node Name.vi"("Name"="SensorIDs", "Attributes"=w978) -> ("Value"=w973:string)  [unwired: 9 in]
                      n302 = call "Read Node Name.vi"("Name"="NumberOfSensors", "Attributes"=w978) -> ("Value"=w975:string)  [unwired: 9 in]
                      n303 = Decimal String To Number(string=w975) -> (number=w974:i32)  [unwired: 2 in, 1 out]
                      n304 = for {
                        N: w974 -> [_]
                        tunnel: w973 -> [w994]
                        shift-right: [w984] -> w971
                        shift-left: w972 -> [w983]
                        tunnel: w970 -> [w982]
                        tunnel: [w981] -> w969
                        i -> [w993]
                        n305 = Multiply(x=w993, y=2) -> (x*y=w991:i32)
                        n306 = String Subset(string=w994, offset (0)=w991, length (rest)=1) -> (substring=w989:string)
                        n307 = call "Find Sensor By ID.vi"("error in (no error)"=w982, "Sensor ID"=w989, "Vessel in"=w983) -> ("error out"=w980:errorcluster, "Sensor Index"=w987:i32, "Vessel out"=w988:refnum<class "Vessel.lvclass">)  [unwired: 6 in]
                        n308 = call "Read Element of Available Sensors.vi"("error in (no error)"=w980, "index"=w987, "Vessel in"=w988) -> ("error out"=w979:errorcluster, "Sensor.lvclass"=w986:refnum<class "Sensor.lvclass">, "Vessel out"=w985:refnum<class "Vessel.lvclass">)  [unwired: 6 in]
                        n309 = call "Add Element in Used Sensors.vi"("error in (no error)"=w979, "Sensor In"=w986, "Vessel in"=w985) -> ("error out"=w981:errorcluster, "Vessel out"=w984:refnum<class "Vessel.lvclass">)  [unwired: 7 in]
                      }
                    }
                    frame "#~", Default {
                    }
                  }
                }
              }
            }
          }
        }
      }
    }
    frame "~" {
    }
  }
  "Vessel Out" <- w11
  "error out" <- w8
  "Controller Names" <- w3
  "Observer Names" <- w1
